vi "Main.vi"(11 "Module Admin":refnum<class "Delacor_lib_QMH_Module Admin.lvclass">) -> ()   [LabVIEW 2019, in "Panther Dashboard.lvlib"]
doc: "Panther Dashboard For DQMH®\n\nDeveloped and maintained by:\nPantherLAB\n\nMain Contributor- Developer:\n\n» Enrique Noé Arias\n\nBrainstorming & Code Reviews:\n\n» Matthias Baudot\n» Fabiola De La Cueva\n» Christopher Farmer\n» Cyril Gambini\n» Joerg Hampel\n» Olivier Jourdan\n» Cesar Muñoz\n» Darren Nattinger\n» Luis Orozco\n» Sam Taggart\n» Diego Torres"
uses:
  Panther Dashboard.lvlib
  <vilib>/Delacor/Delacor QMH/Libraries/Module Admin_class/Delacor_lib_QMH_Module Admin.lvclass
  Module Data--cluster.ctl
  Maps List and refs--cluster.ctl
  <vilib>/National Instruments/Tree Map/Tree Map Data.ctl
  DQMH Modules Info--cluster.ctl
  Module type--enum.ctl
  Project References--cluster.ctl
  Selection Type--enum.ctl
  References Updated Argument--cluster.ctl
  Launch DQMH Scripting Tools Argument--cluster.ctl
  DQMH Tools Menu--enum.ctl
  <vilib>/Delacor/Delacor QMH/Libraries/Message Queue_class/Delacor_lib_QMH_Message Queue.lvclass/Delacor_lib_QMH_Message Queue.ctl
  Expand Results Argument--cluster.ctl
  Execute Default Event Request Argument--cluster.ctl
  Tree DQMH Selection Argument--cluster.ctl
  Scan DQMH Modules Argument--cluster.ctl
  Stop Argument--cluster.ctl
  Generate Project Documentation Argument--cluster.ctl
  Set App Theme Argument--cluster.ctl
  Show About Argument--cluster.ctl
  Update Module ID Argument--cluster.ctl
  Save Library Description Argument--cluster.ctl
  Save VI Description Argument--cluster.ctl
  Open Documentation Argument--cluster.ctl
  Save Project Documentation Argument--cluster.ctl
  <vilib>/Delacor/Delacor QMH/Libraries/Module Admin_class/Delacor_lib_QMH_Module Admin.lvclass/Delacor_lib_QMH_Module Admin.ctl
  <vilib>/Delacor/Delacor QMH/Libraries/Message Queue_class/Delacor_lib_QMH_Enqueue Message (Single).vi
  <vilib>/Delacor/Delacor QMH/Libraries/Module Admin_class/Delacor_lib_QMH_Get External Launch.vi
  Panther Dashboard--global.vi
  <vilib>/National Instruments/Tree Map/API/List Roots.vi
  <vilib>/National Instruments/Tree Map/Utility/Into Tree Control Items.vi
  <vilib>/Platform/browser.llb/Open URL in Default Browser (path).vi
  <vilib>/Utility/error.llb/Error Cluster From Error Code.vi
  <vilib>/ErrorRing/Error Ring.xnode
  <vilib>/Delacor/Delacor QMH/Libraries/Message Queue_class/Delacor_lib_QMH_Message Queue.lvclass
  <vilib>/National Instruments/Tree Map/Tree Map.lvlib
  <vilib>/Delacor/Delacor QMH/Libraries/Scripting API/DQMH_Scripting API.lvlib
  Shared/Shared.lvlib
  ContextHelp/ContextHelp.lvlib
panel:
  out "error out":errorcluster
  in  "Add Event":bool
  in  "Remove Event":bool caption="Remove"
  in  "Convert Event":bool caption="Convert"
  in  "Rename Event":bool caption="Rename"
  in  "Add New Module":bool caption="Add"
  in  "Rename Module":bool caption="Rename"
  in  "Validate Module":bool caption="Validate"
  in  "Create Module Template":bool caption="Template"
  in  "Add Unit Test Module":bool caption="Unit Test"
  in  "Create RT Tester Module":bool caption="RT Tester"
  in  "Open Antidoc Output":bool caption="Open"
  in  "Generate Antidoc":bool caption="Antidoc"
  in  "About Panther":bool caption="About"
  in  "Theme Panther":bool caption="Theme"
  in  "Projects":string(combo)
  in  "Targets":string(combo)
  in  "Doc Editor":bool
  in  "Search":bool caption="Scan Project"
  in  "Expand Results":bool
  in  "Include Dependencies":bool
  in  "Module ID":i32=-1 min=-1 max=1000 step=1 format="Module ID %d"
  in  "Modules Tree":string(tree) caption="Tree 2"
  out "antidoc":bool
  out "Panther Indicator":bool
  out "Process Indicator":bool
  out "Event Indicator":bool
  out "Status":string
  out "Progress":u16(slide) scale=0.0..1.0
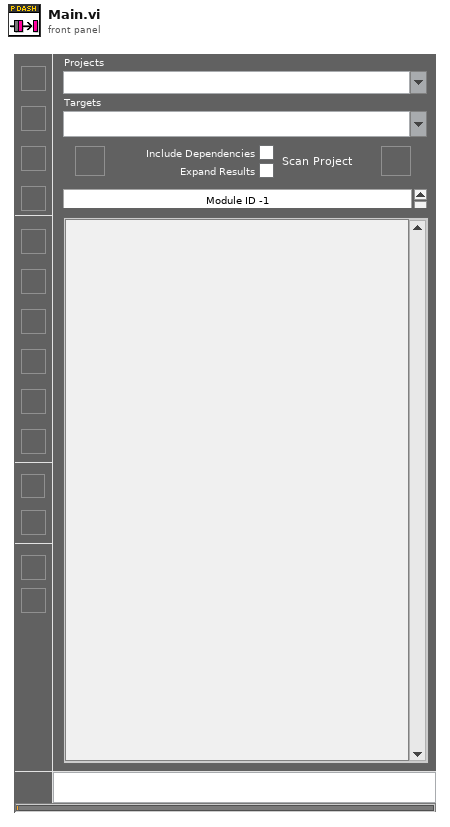
[diagram p1: front panel]
types:
  T1 = typedef "Panther Dashboard.lvlib/Broadcast Events--cluster.ctl" = cluster{"Module Did Init":refnum<user-event>, "Status Updated":refnum<user-event>, "Error Reported":refnum<user-event>, "Module Did Stop":refnum<user-event>, "Update Module Execution Status":refnum<user-event>, "References Updated":refnum<user-event>, "Projects Updated":refnum<user-event>, "Targets Updated":refnum<user-event>, "Progress updated":refnum<user-event>, "Scale Updated":refnum<user-event>, "Connector Pane Updated":refnum<user-event>, "Documentation Updated":refnum<user-event>, "Module Type Updated":refnum<user-event>, "Theme Updated":refnum<user-event>, "Project Description Updated":refnum<user-event>}
  T2 = typedef "Panther Dashboard.lvlib/Request Events--cluster.ctl" = cluster{"Stop Module":refnum<user-event>, "Show Panel":refnum<user-event>, "Hide Panel":refnum<user-event>, "Get Module Execution Status":refnum<user-event>, "Show Diagram":refnum<user-event>, "Scan DQMH Modules":refnum<user-event>, "Tree DQMH Selection":refnum<user-event>, "Open Module API Tester":refnum<user-event>, "Execute Default Event Request":refnum<user-event>, "Expand Results":refnum<user-event>, "Launch DQMH Scripting Tools":refnum<user-event>, "Generate Project Documentation":refnum<user-event>, "Set App Theme":refnum<user-event>, "Show About":refnum<user-event>, "Update Module ID":refnum<user-event>, "Save Library Description":refnum<user-event>, "Save VI Description":refnum<user-event>, "Open Documentation":refnum<user-event>, "Save Project Documentation":refnum<user-event>, "Register controls Mouse Enter":refnum<user-event>}
  T3 = typedef "ContextHelp.lvlib/Broadcast Events--cluster.ctl" = cluster{"Module Did Init":refnum<user-event>, "Status Updated":refnum<user-event>, "Error Reported":refnum<user-event>, "Module Did Stop":refnum<user-event>, "Update Module Execution Status":refnum<user-event>}
  T4 = typedef "Panther Dashboard.lvlib/Selection Type--enum.ctl" = enum16{"Broadcast", "Request", "Module", "Public API"}
  T5 = typedef "Panther Dashboard.lvlib/Module Data--cluster.ctl" = cluster{"Maps":T6, "DQMH Scan Results":T8, "Current Selection":cluster{"VI Ref":refnum<vi>, "DQMH Lib Ref":refnum<vi>}, "Module type":T9, "Module ID":i32, "Theme":bool, "Broadcast?":bool}
  T6 = typedef "Panther Dashboard.lvlib/Maps List and refs--cluster.ctl" = cluster{"Tree Map":T7, "References Map":map{string, refnum<vi>}}
  T7 = typedef "Tree Map.lvlib/Tree Map Data.ctl" = map{string, cluster{"Child Paths Set":set{string}, "Name":string, "Data":string, "Attributes":map{string, string}}}
  T8 = typedef "Panther Dashboard.lvlib/DQMH Modules Info--cluster.ctl" = cluster{"All DQMH Modules Refs":refnum<vi>[], "All Modules Descriptions":string[], "All Modules type":T9[], "Project References":T10}
  T9 = typedef "Panther Dashboard.lvlib/Module type--enum.ctl" = enum16{"Module type: Singleton", "Module type: Cloneable"}
  T10 = typedef "Panther Dashboard.lvlib/Project References--cluster.ctl" = cluster{"Project Ref":refnum<vi>, "Project Name":string, "Target":refnum<vi>, "App Ref":refnum<vi>}
  T11 = typedef "Panther Dashboard.lvlib/References Updated Argument--cluster.ctl" = cluster{"Modules":refnum<vi>[], "Modules Types":T9[], "Application Instance":refnum<vi>}
  T12 = enum8{"Enabled", "Disabled", "Disabled and Grayed Out"}
  T13 = typedef "Panther Dashboard.lvlib/Launch DQMH Scripting Tools Argument--cluster.ctl" = cluster{"Scripting Tool":T14}
  T14 = typedef "Panther Dashboard.lvlib/DQMH Tools Menu--enum.ctl" = enum16{"Create New DQMH Event", "Remove DQMH Event", "Convert DQMH Event", "Rename DQMH Event", "Add New DQMH Module", "Create RT Tester", "Rename DQMH Module", "Validate DQMH Module", "Create DQMH Module Template", "New DQMH  Unit Test"}
  T15 = typedef "Panther Dashboard.lvlib/Expand Results Argument--cluster.ctl" = cluster{"Expand?":bool}
  T16 = typedef "Panther Dashboard.lvlib/Execute Default Event Request Argument--cluster.ctl" = cluster{"Event Name":string}
  T17 = typedef "Panther Dashboard.lvlib/Tree DQMH Selection Argument--cluster.ctl" = cluster{"Tree DQMH Sel":string}
  T18 = typedef "Panther Dashboard.lvlib/Scan DQMH Modules Argument--cluster.ctl" = cluster{"Include Dependencies":bool, "Project":string, "Target":string}
  T19 = enum32{"invalid lock state", "Not Locked", "Locked (No Password)", "Password-protected"}
  T20 = typedef "Panther Dashboard.lvlib/Stop Argument--cluster.ctl" = cluster{"Origin":string, "Exit via Stop Module Req?":bool, "Wait for Module to stop?":bool}
  T21 = typedef "Panther Dashboard.lvlib/Generate Project Documentation Argument--cluster.ctl" = cluster{"Boolean":bool}
  T22 = typedef "Panther Dashboard.lvlib/Set App Theme Argument--cluster.ctl" = cluster{"Theme":bool}
  T23 = typedef "Panther Dashboard.lvlib/Show About Argument--cluster.ctl" = cluster{"Boolean":bool}
  T24 = typedef "Panther Dashboard.lvlib/Update Module ID Argument--cluster.ctl" = cluster{"New ID":i32}
  T25 = typedef "Panther Dashboard.lvlib/Save Library Description Argument--cluster.ctl" = cluster{"Library Description":string}
  T26 = typedef "Panther Dashboard.lvlib/Save VI Description Argument--cluster.ctl" = cluster{"VI Description":string}
  T27 = typedef "Panther Dashboard.lvlib/Open Documentation Argument--cluster.ctl" = cluster{"Boolean":bool}
  T28 = typedef "Panther Dashboard.lvlib/Save Project Documentation Argument--cluster.ctl" = cluster{"Project Description":string}
  T29 = cluster{"Left Cell String":string, "Child Text":string[], "Child Tag":string, "Item Indent":i32, "Child Only?":bool, "Glyph Index":i32}[]
  T30 = typedef "LVRectTypeDef.ctl" = cluster{"Left":i16, "Top":i16, "Right":i16, "Bottom":i16}
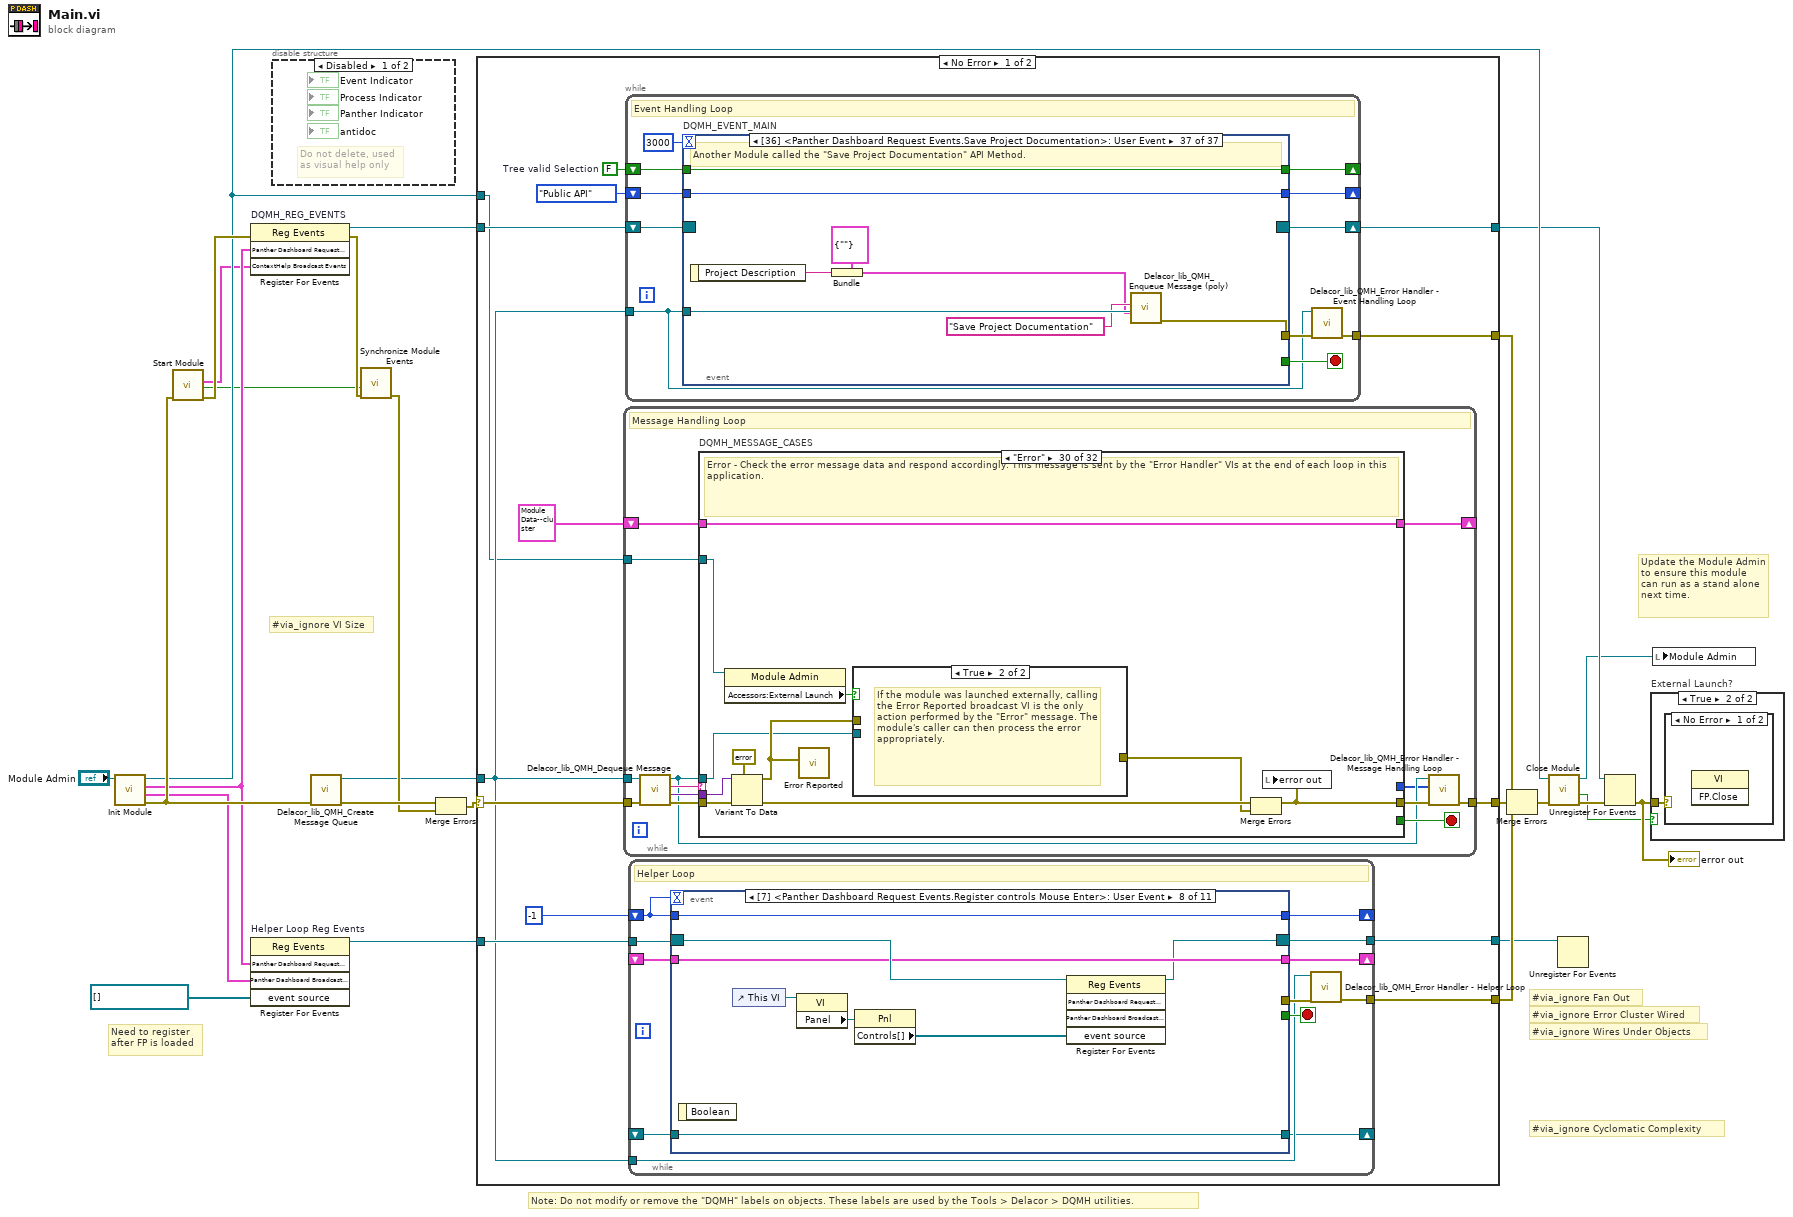
[diagram p0: block diagram]
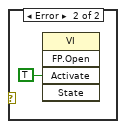
[diagram p4: hidden frame]
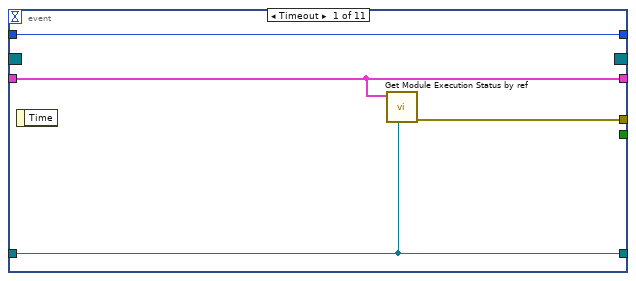
[diagram p5: hidden frame]
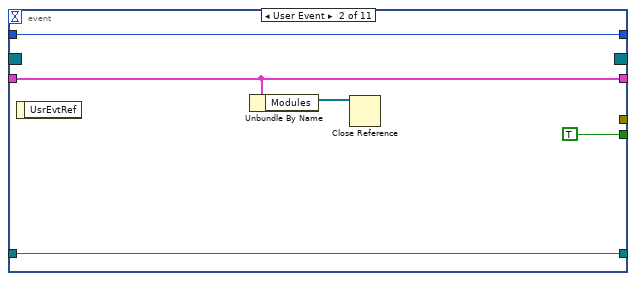
[diagram p6: hidden frame]
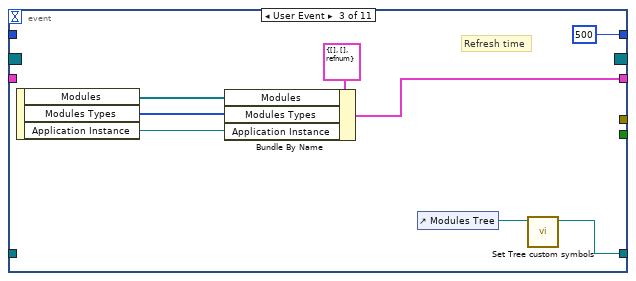
[diagram p7: hidden frame]
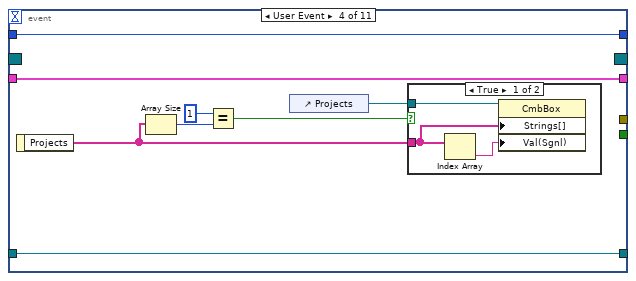
[diagram p8: hidden frame]
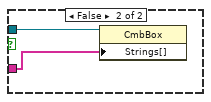
[diagram p9: hidden frame]
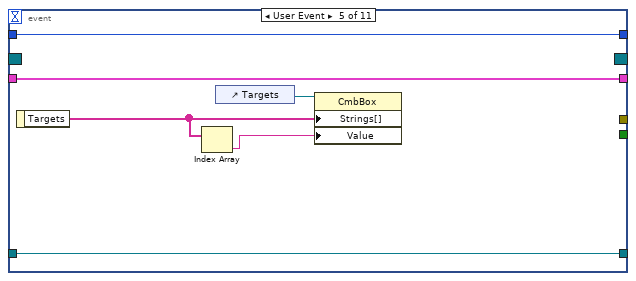
[diagram p10: hidden frame]
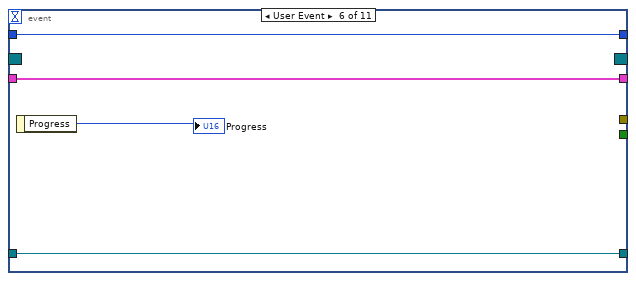
[diagram p11: hidden frame]
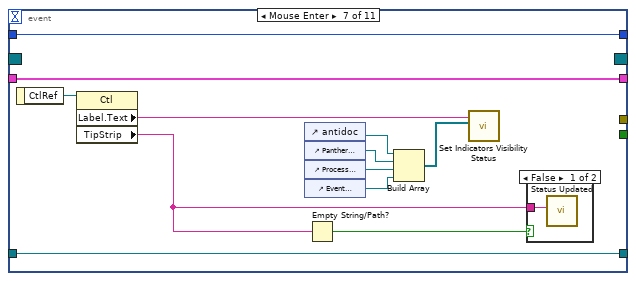
[diagram p12: hidden frame]
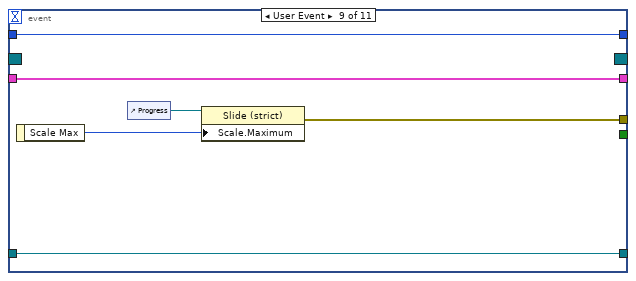
[diagram p14: hidden frame]
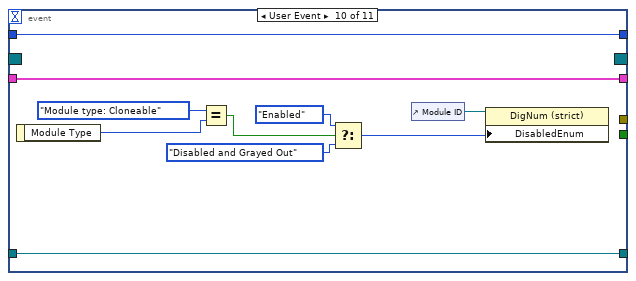
[diagram p15: hidden frame]
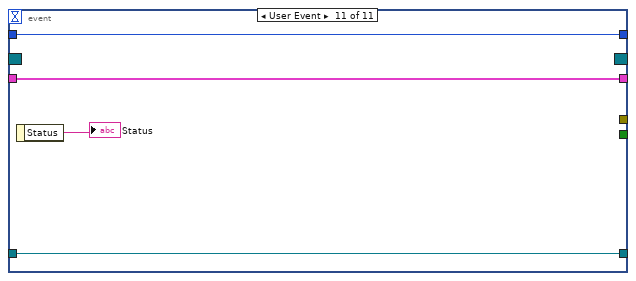
[diagram p16: hidden frame]
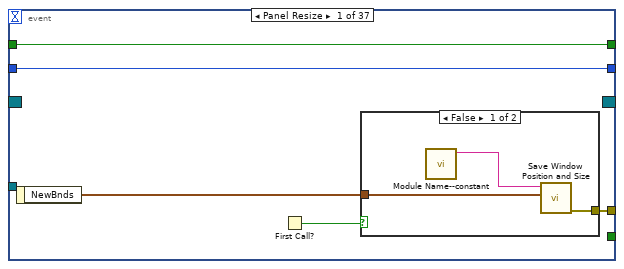
[diagram p17: hidden frame]
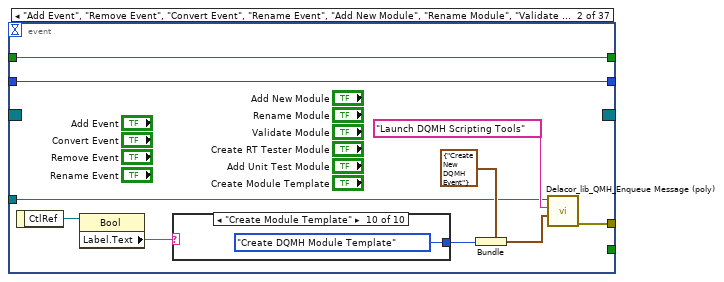
[diagram p19: hidden frame]
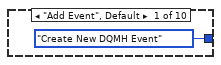
[diagram p20: hidden frame]
diagram:
  # "Need to register\nafter FP is loaded"
  # "#via_ignore VI Size"
  # "#via_ignore Fan Out"
  # "#via_ignore Cyclomatic Complexity"
  # "#via_ignore Wires Under Objects"
  # "#via_ignore Error Cluster Wired"
  # "Note: Do not modify or remove the \"DQMH\" labels on objects. These labels are used by the Tools > Delacor > DQMH utilities."
  # "Update the Module Admin to ensure this module can run as a stand alone next time."
  n1 = call "Init Module.vi"("Singleton Module Admin in"="Module Admin") -> ("error out"=w15:errorcluster, "Panther Dashboard Broadcast Events"=w4:T1, "Panther Dashboard Request Events"=w5:T2, "Singleton Module Admin out"=w14:refnum<class "Delacor_lib_QMH_Module Admin.lvclass">)  [unwired: 7 in]
  n2 = call "Start Module.vi"("error in"=w15) -> ("error out"=w17:errorcluster, "Wait for Event Sync?"=w3:bool, "ContextHelp Broadcast Events"=w2:T3)  [unwired: 7 in, 1 out]
  n3 = register-events "DQMH_REG_EVENTS"(error in=w17, w5, w2) -> (reference out=w12:refnum<event-registration>, error out=w18:errorcluster)  [unwired: 1 in]
  n4 = register-events "Helper Loop Reg Events"(w5, w4, refnum<vi>[] [] ("event source")) -> (reference out=w7:refnum<event-registration>)  [unwired: 2 in, 1 out]
  n5 = disable-structure shown="Disabled" {
    frame Disabled {
      # "Do not delete, used\nas visual help only"
    }
    frame Enabled {
    }
  }
  n6 = call <vilib>:"Delacor_lib_QMH_Create Message Queue.vi"("error in"=w15) -> ("error out"=w21:errorcluster, "Message Queue"=w11:refnum<class "Delacor_lib_QMH_Message Queue.lvclass">)  [unwired: 9 in]
  n7 = call "Synchronize Module Events.vi"("error in"=w18, "Wait for Event Sync?"=w3) -> ("error out"=w16:errorcluster)  [unwired: 9 in]
  n8 = Merge Errors(w21, w16) -> (w20:errorcluster)
  n9 = case shown="No Error" w20 {
    selector: w20 -> [w38 w815]
    tunnel: [w40 w814] -> w26
    tunnel: [w36 w813] -> w13
    tunnel: w12 -> [w34 w813]
    tunnel: w11 -> [w30 w809]
    tunnel: [w39 _] -> w24
    tunnel: w14 -> [w27 w810]
    tunnel: w7 -> [w33 w808]
    tunnel: [w32 w808] -> w6
    tunnel: [w37 _] -> w19
    frame No Error {
      w29 = FALSE  # Tree valid Selection
      n10 = while {
        tunnel: w30 -> [w458]
        shift-right: [w462] -> _
        shift-left: T5 {"Maps"={"Tree Map"={}, "References Map"={}}, "DQMH Scan Results"={"All DQMH Modules Refs"=[], "All Modules Descriptions"=[], "All Modules type"=[], "Project References"={"Project Ref"=refnum, "Project Name"="", "Target"=refnum, "App Ref"=refnum}}, "Current Selection"={"VI Ref"=refnum, "DQMH Lib Ref"=refnum}, "Module type"=enum."Module type: Singleton", "Module ID"=0, "Theme"=FALSE, "Broadcast?"=FALSE} ("Data Cluster") -> [w463]
        tunnel: w38 -> [w466]
        tunnel: [w464] -> w40
        tunnel: w27 -> [w456]
        stop <- w461 stop-if-true
        # "Message Handling Loop"
        n11 = call-dynamic "Delacor_lib_QMH_Dequeue Message.vi"("error in"=w466, "Message Queue in"=w458) -> ("error out"=w465:errorcluster, "Message Data"=w459:variant, "Message"=w460:string, "Message Queue out"=w457:refnum<class "Delacor_lib_QMH_Message Queue.lvclass">)  [unwired: 6 in]
        n12 = case "DQMH_MESSAGE_CASES" shown="\"Error\"" w460 {
          selector: w460 -> [_ w491 _ _ _ _ _ _ _ _ _ _ _ _ _ _ _ _ _ _ _ _ _ _ _ _ _ _ _ _ _ w794]
          tunnel: w457 -> [_ _ _ _ _ _ _ _ _ _ _ _ _ _ _ _ _ _ _ _ _ _ _ _ _ _ _ _ _ w760 w786 _]
          tunnel: w465 -> [w488 w496 w498 w519 w526 w533 w540 w555 w564 w569 w575 w589 w602 w624 w630 w637 w644 w649 w662 w671 w682 w691 w699 w709 w725 w741 w752 w755 w757 w767 w792 w796]
          tunnel: [w482 w494 w498 w518 w525 w533 w540 w554 w563 w570 w576 w587 w600 w625 w629 w636 w643 w648 w660 w669 w672 w687 w698 w707 w723 w740 w750 w754 w757 w763 w789 w797] -> w467
          tunnel: w463 -> [w479 w493 w497 w505 w523 w531 w539 w550 w562 w568 w574 w582 w599 w623 w628 w635 w642 w647 w651 w665 w679 w686 w697 w701 w718 w730 w746 w753 w756 w762 w778 w795]
          tunnel: [w478 w493 w497 w510 w523 w531 w539 w546 w562 w568 w574 w582 w599 w623 w628 w633 w642 w647 w651 w665 w674 w686 w693 w700 w716 w730 w746 w753 w756 w762 w778 w795] -> w462
          tunnel: [_ _ _ _ _ _ _ _ _ _ _ _ _ _ _ _ _ _ _ _ _ _ _ _ _ _ _ _ _ _ w785 _] -> w461
          tunnel: w459 -> [_ w492 _ w513 _ _ _ w553 _ _ _ w585 _ _ _ w634 w641 _ w659 w667 w678 w685 w696 w705 w721 w739 w749 _ _ w761 w784 _]
          tunnel: w456 -> [w480 _ _ _ _ _ _ _ _ _ _ _ _ _ _ _ _ _ _ _ _ _ _ _ _ _ _ _ _ w759 w779 _]
          tunnel: [_ _ _ _ _ _ _ _ _ _ _ _ i32[] [5000, 1026, 43] ("specific error code to clear (0: all)") _ _ _ _ _ _ _ _ _ _ _ _ _ _ _ _ _ _ _] -> w455
          frame "Initialize" {
            w469 = "Panther Dashboard for DQMH" ("format string")
            # "Initialize - Any operation that needs to be done before the module can receive messages. Synchronize Caller Events.vi will inform Start Module.vi that the module has launched and is ready to receive messages. Module Did Init.vi will broadcast that the module initialized."
            n13 = call "Synchronize Caller Events.vi"("error in (no error)"=w488, "Singleton Module Admin in"=w480) -> ("error out"=w487:errorcluster)  [unwired: 8 in, 1 out]
            n14 = invoke on="Modules Tree" class="Tree (strict)" method="Edit Tree Items.Delete"() -> ()  [unwired: 5 in, 5 out]
            n15 = property on="Modules Tree" class="Tree (strict)"("Allow Item Drag"=TRUE ("Drag/Drop:Allow Dragging"), "SelColor"=u32 8355711) -> ()  [unwired: 2 in, 2 out]
            n16 = call "Module Name--constant.vi"() -> ("Module Name"=w476:string)  [unwired: 11 in]
            n17 = call "Module Did Init.vi"("error in (no error)"=w487, "Initialized?"=TRUE, "Origin"=w476) -> ("error out"=w486:errorcluster)  [unwired: 8 in]
            n18 = control-ref of="Projects"() -> (w472:refnum<vi>)
            n19 = call "Scan For App Projects.vi"("error in"=w486, "Init?"=TRUE, "Projects Ref"=w472) -> ("error out"=w485:errorcluster)  [unwired: 8 in]
            n20 = call "Read Theme from Config.vi"("error in"=w485) -> ("error out"=w484:errorcluster, "Theme"=w468:bool)  [unwired: 9 in]
            n21 = local write "Theme Panther"(w468) -> ()
            n22 = call "Set App Theme.vi"("error in"=w484, "Theme"=w468) -> ("error out"=w483:errorcluster)  [unwired: 9 in]
            n23 = control-ref of="This VI"() -> (w470:refnum<vi>)
            n24 = Bundle By Name(cluster=w479, "Module ID"=-1) -> (w478:T5)
            n25 = call "Status Updated.vi"("Status"=w469) -> ()  [unwired: 10 in, 1 out]
            n26 = call "Set Panel Initial State.vi"("Title"=w469, "Main Vi Ref"=w470) -> ("error out"=w481:errorcluster)  [unwired: 9 in]
            n27 = Merge Errors(w481, w483) -> (w482:errorcluster)
          }
          frame "Refresh Targets" {
            # "When the User selects a Project triggers this task to scan all the targets available"
            n28 = Variant To Data(error in=w496, type=w491, Variant=w492) -> (data=w490:string, error out=w495:errorcluster)
            n29 = call "Get all Targets.vi"("error in"=w495, "Project Selection"=w490) -> ("error out"=w494:errorcluster, "Targets"=w489:string[])  [unwired: 8 in]
            n30 = call "Targets Updated.vi"("Targets"=w489) -> ()  [unwired: 10 in, 1 out]
          }
          frame "---Module Specific---" {
            # "Separator -- The following cases handle messages specific to this Module."
          }
          frame "Scan DQMH Modules" {
            # "Scan DQMH Modules in the project and fill 2 maps one with the Vi References and the another one with the list of DQMH modules on the project"
            n31 = Variant To Data(error in=w519, type=T18 {"Include Dependencies"=FALSE, "Project"="", "Target"=""} ("Scan DQMH Modules Argument"), Variant=w513) -> (data=w511:T18, error out=w516:errorcluster)
            n32 = call "Close vi references.vi"("Data Cluster"=w505) -> ("error out"=w515:errorcluster)  [unwired: 10 in]
            n33 = Unbundle By Name(w511) -> ("Project"=w501:string, "Target"=w503:string, "Include Dependencies"=w504:bool)
            n34 = invoke on="Modules Tree" class="Tree (strict)" method="Edit Tree Items.Delete"(error in=w515, "Delete Children"=TRUE ("Delete Children?")) -> (error out=w514:errorcluster)  [unwired: 3 in, 4 out]
            n35 = local write "Include Dependencies"(w504) -> ()
            n36 = call <vilib>:"Set Busy.vi"("error in (no error)"=w514) -> ()  [unwired: 9 in, 2 out]
            n37 = call "Scan DQMH Modules and create Maps.vi"("error in"=w516, "Include Dependencies"=w504, "Target Selection"=w503, "Project"=w501) -> ("error out"=w518:errorcluster, "Tree Map out"=w502:T7, "map ref out"=w506:map{string, refnum<vi>}, "DQMH Scan Results"=w509:T8)  [unwired: 4 in]
            n38 = control-ref of="Modules Tree"() -> (w507:refnum<vi>)
            n39 = call <vilib>:"Tree Map to Tree Control Items.vi"("Tree Map In"=w502) -> ("Tree Control Items"=w508:T29)  [unwired: 10 in]
            n40 = Bundle By Name(cluster=w505, "DQMH Scan Results"=w509, "Maps.References Map"=w506, "Maps.Tree Map"=w502) -> (w510:T5)
            n41 = local read "Expand Results"() -> (w499:bool)
            n42 = call "Draw Tree.vi"("Expanded Results?"=w499, "Tree Control Items"=w508, "TreeControl in"=w507) -> ("error out"=w517:errorcluster)  [unwired: 8 in]
            n43 = call <vilib>:"Unset Busy.vi"("error in (no error)"=w517) -> ()  [unwired: 10 in, 1 out]
          }
          frame "Drag VI" {
            # "This is the functionality alowing drag and drop the current selection to your code, you can build code using panther Dashboard."
            n44 = Unbundle By Name(w523) -> ("DQMH Scan Results.Project References.App Ref"=w522:refnum<vi>, "DQMH Scan Results.Project References.Target"=w521:refnum<vi>, "Current Selection.VI Ref"=w520:refnum<vi>)
            n45 = call "Drop Event into subVI.vi"("Current Selection.VI Ref"=w520, "Target"=w521, "App Ref"=w522) -> ("error out"=w524:errorcluster)  [unwired: 8 in]
            n46 = Merge Errors(w524, w526) -> (w525:errorcluster)
          }
          frame "Who is launching this module?" {
            w532 = 0  # Start Module.vi index
            # "Find all the VIS calling the Start Module.vi of the selected module library"
            n47 = Unbundle By Name(w531) -> ("Theme"=w530:bool, "DQMH Scan Results.Project References.App Ref"=w529:refnum<vi>, "DQMH Scan Results.Project References.Target"=w528:refnum<vi>, "Current Selection.DQMH Lib Ref"=w527:refnum<vi>)
            n48 = call "Find some Public API VI.vi"("Theme"=w530, "Public Api file index"=w532, "Library in"=w527, "Target"=w528, "App Ref"=w529) -> ()  [unwired: 7 in]
          }
          frame "Who is registered to this module's broadcasts?" {
            w538 = 2  # Obtain Broadcast Events for Registration.vi index
            # "Find all the VIS calling the Obtain broadcast events for registration of the selected module library"
            n49 = Unbundle By Name(w539) -> ("Theme"=w537:bool, "DQMH Scan Results.Project References.App Ref"=w536:refnum<vi>, "DQMH Scan Results.Project References.Target"=w535:refnum<vi>, "Current Selection.DQMH Lib Ref"=w534:refnum<vi>)
            n50 = call "Find some Public API VI.vi"("Theme"=w537, "Public Api file index"=w538, "Library in"=w534, "Target"=w535, "App Ref"=w536) -> ()  [unwired: 7 in]
          }
          frame "Tree DQMH Selection" {
            # "There is a new selection of the DQMH Tree list, need to search and update indicators acordanly."
            n51 = Unbundle By Name(w550) -> ("Maps.Tree Map"=w549:T7, "Maps.References Map"=w548:map{string, refnum<vi>}, "DQMH Scan Results"=w547:T8)
            n52 = Variant To Data(error in=w555, type=T17 {"Tree DQMH Sel"=""} ("Tree DQMH Selection Argument"), Variant=w553) -> (data=w551:T17, error out=w554:errorcluster)
            n53 = Unbundle By Name(w551) -> ("Tree DQMH Sel"=w543:string)
            n54 = call "Get List Information.vi"("List Selection"=w543, "DQMH Scan Info"=w547, "References Map"=w548, "Tree Map"=w549) -> ("Broadcast?"=w541:bool, "Vi out"=w544:refnum<vi>, "Module type"=w542:T9, "DQMH Lib"=w545:refnum<vi>)  [unwired: 4 in]
            n55 = Bundle By Name(cluster=w550, "Current Selection.DQMH Lib Ref"=w545, "Current Selection.VI Ref"=w544, "Module type"=w542, "Broadcast?"=w541) -> (w546:T5)
          }
          frame "Open Module API Tester" {
            # "If nothing selected use the first DQMH module"
            # "Open the API Tester from the current DQMH Module Selected"
            n56 = Unbundle By Name(w562) -> ("DQMH Scan Results.Project References.App Ref"=w561:refnum<vi>, "DQMH Scan Results.All DQMH Modules Refs"=w560:refnum<vi>[], "Current Selection.DQMH Lib Ref"=w556:refnum<vi>)
            n57 = Index Array(array=w560) -> (element=w558:refnum<vi>)  [unwired: 1 in]
            n58 = Not A Number/Path/Refnum?(number/path/refnum=w556) -> (NaN/Path/Refnum?=w559:bool)
            n59 = Select(t=w558, s=w559, f=w556) -> (s? t:f=w557:refnum<vi>)
            n60 = call "Open API Tester.vi"("error in"=w564, "DQMH Library Ref"=w557, "Application Instance"=w561) -> ("error out"=w563:errorcluster)  [unwired: 8 in]
          }
          frame "Find Module in project" {
            # "Find the selected module in project explorer"
            n61 = Unbundle By Name(w568) -> ("Current Selection.DQMH Lib Ref"=w567:refnum<vi>, "DQMH Scan Results.Project References.Project Ref"=w566:refnum<vi>, "DQMH Scan Results.All DQMH Modules Refs"=w565:refnum<vi>[])
            n62 = call "Find Library in Project.vi"("error in (no error)"=w569, "DQMH Modules Refs"=w565, "Project Ref"=w566, "DQMH Lib Ref"=w567) -> ("error out"=w570:errorcluster)  [unwired: 7 in]
          }
          frame "Locate Event on Main" {
            # "Find the selected event vi on the owing DQMH Module, if it is a reques we highlight its frame, if it is a broadcast we highlight where the broadcast is being triggered"
            n63 = Unbundle By Name(w574) -> ("DQMH Scan Results.Project References.App Ref"=w572:refnum<vi>, "Current Selection.VI Ref"=w573:refnum<vi>, "Broadcast?"=w571:bool)
            n64 = call "Find Event Frame.vi"("error in"=w575, "Broadcast?"=w571, "VI in"=w573, "Application Instance"=w572) -> ("error out"=w576:errorcluster)  [unwired: 7 in]
          }
          frame "Execute Default Event Request" {
            # "Execute Default Event"
            n65 = Variant To Data(error in=w589, type=T16 {"Event Name"=""} ("Execute Default Event Request Argument"), Variant=w585) -> (data=w583:T16, error out=w588:errorcluster)
            n66 = Unbundle By Name(w582) -> ("DQMH Scan Results.Project References.App Ref"=w581:refnum<vi>, "Current Selection.DQMH Lib Ref"=w580:refnum<vi>, "Module ID"=w578:i32, "Module type"=w577:T9)
            n67 = Unbundle By Name(w583) -> ("Event Name"=w579:string)
            n68 = call "Execute Default event.vi"("Module type"=w577, "Module ID"=w578, "Event"=w579, "DQMH Library Ref"=w580, "application Instance"=w581) -> ("error out"=w586:errorcluster)  [unwired: 6 in]
            n69 = Merge Errors(w588, w586) -> (w587:errorcluster)
          }
          frame "Search for Event Callers / listeners" {
            # "1026-Invalid Ref\n43- Operation\n canceled by user\n5000- something\nrandom happening\non DQMH Scripting\nAPI"
            # "Search for this event callers"
            n70 = Unbundle By Name(w599) -> ("DQMH Scan Results.Project References.Project Ref"=w593:refnum<vi>, "Current Selection.VI Ref"=w598:refnum<vi>, "Theme"=w590:bool, "Broadcast?"=w591:bool)
            n71 = Select(t="Searching code registered to broadcast selection" ("Status"), s=w591, f="Searching for Event Callers" ("Status")) -> (s? t:f=w594:string)
            n72 = call "Status Updated.vi"("error in (no error)"=w602, "Status"=w594) -> ("error out"=w601:errorcluster)  [unwired: 9 in]
            n73 = case shown="False" w591 {
              tunnel: w601 -> [w607 w614]
              tunnel: [w606 w613] -> w600
              tunnel: w598 -> [w605 w610]
              tunnel: [w604 w612] -> w597
              tunnel: w593 -> [w603 w611]
              frame False {
                # "Requests"
                n74 = call <vilib>:"Get Callers of Request VI in Project.vi"("error in"=w607, "Request VI"=w605, "Project"=w603) -> ("error out"=w606:errorcluster, "Request VI Callers"=w604:refnum<vi>[])  [unwired: 7 in]
              }
              frame True {
                # "Broadcast"
                n75 = Two Button Dialog(message="This is an exhaustive task that can take up to minutes, do you wish to continue?") -> (T button?=w609:bool)  [unwired: 2 in]
                n76 = case shown="False" w609 {
                  tunnel: w614 -> [w615 w620]
                  tunnel: [w615 w619] -> w613
                  tunnel: [_ w618] -> w612
                  tunnel: w611 -> [_ w617]
                  tunnel: w610 -> [_ w616]
                  frame False {
                  }
                  frame True {
                    n77 = call <vilib>:"Get VIs Registered for Broadcast in Project.vi"("error in"=w620, "Broadcast VI"=w616, "Project"=w617) -> ("error out"=w619:errorcluster, "VIs Registered for Broadcast"=w618:refnum<vi>[])  [unwired: 7 in]
                  }
                }
              }
            }
            n78 = call <vilib>:"Set Busy.vi"("error in (no error)"=w601) -> ()  [unwired: 9 in, 2 out]
            n79 = call <vilib>:"Unset Busy.vi"("error in (no error)"=w600) -> ()  [unwired: 10 in, 1 out]
            n80 = call "Start Call to results window.vi"("Find Broadcast?"=w591, "Request VI Callers"=w597, "Event"=w598, "Theme"=w590) -> ()  [unwired: 8 in]
          }
          frame "Open VI on Disk" {
            # "Open current event selection on the file system"
            n81 = Unbundle By Name(w623) -> ("Current Selection.VI Ref"=w622:refnum<vi>)
            n82 = property class="VI"(reference=w622) -> ("Path"=w621:path)  [unwired: 1 in, 2 out]
            n83 = call "Open File on Disk.vi"("error in"=w624, "file or directory path"=w621) -> ("error out"=w625:errorcluster)  [unwired: 9 in]
          }
          frame "Open File Library on Disk" {
            # "Open current Module Library selection on the file system"
            n84 = Unbundle By Name(w628) -> ("Current Selection.DQMH Lib Ref"=w627:refnum<vi>)
            n85 = property class="Library"(reference=w627) -> ("Path"=w626:path)  [unwired: 1 in, 2 out]
            n86 = call "Open File on Disk.vi"("error in"=w630, "file or directory path"=w626) -> ("error out"=w629:errorcluster)  [unwired: 9 in]
          }
          frame "Module ID Update" {
            # "Module ID Control has value change"
            n87 = Variant To Data(error in=w637, type=0 ("Module ID"), Variant=w634) -> (data=w632:i32, error out=w636:errorcluster)
            n88 = Bundle By Name(cluster=w635, "Module ID"=w632) -> (w633:T5)
          }
          frame "Expand or Close" {
            # "Expand or Close DQMH Tree control"
            n89 = Variant To Data(error in=w644, type=T15 {"Expand?"=FALSE} ("Expand or Close Argument"), Variant=w641) -> (data=w639:T15, error out=w643:errorcluster)
            n90 = Unbundle By Name(w639) -> ("Expand?"=w638:bool)
            n91 = invoke on="Modules Tree" class="Tree (strict)" method="Open/Close.Open/Close All"("Open"=w638) -> ()  [unwired: 3 in, 4 out]
          }
          frame "Open Project Folder" {
            n92 = Unbundle By Name(w647) -> ("DQMH Scan Results.Project References.Project Ref"=w646:refnum<vi>)
            n93 = property class="Project"(reference=w646) -> ("Path"=w645:path)  [unwired: 1 in, 2 out]
            n94 = call "Open File on Disk.vi"("error in"=w649, "file or directory path"=w645) -> ("error out"=w648:errorcluster)  [unwired: 9 in]
          }
          frame "Launch DQMH Scripting Tools" {
            # "Launch the DQMH Scripting Tools"
            n95 = Variant To Data(error in=w662, type=T13 {"Scripting Tool"=enum."Create New DQMH Event"} ("Launch DQMH Scripting Tools Argument"), Variant=w659) -> (data=w657:T13, error out=w661:errorcluster)
            n96 = Unbundle By Name(w657) -> ("Scripting Tool"=w652:T14)
            n97 = Unbundle By Name(w651) -> ("DQMH Scan Results.Project References.Project Name"=w655:string, "DQMH Scan Results.Project References.App Ref"=w656:refnum<vi>, "Current Selection.DQMH Lib Ref"=w650:refnum<vi>)
            n98 = Format Into String(format string="DQMH Tool: %s being executed ", w652) -> (resulting string=w654:string)  [unwired: 2 in, 1 out]
            n99 = call "Status Updated.vi"("Status"=w654) -> ()  [unwired: 10 in, 1 out]
            n100 = call "Launch DQMH Tools by menu.vi"("Project"=w655, "Application Instance"=w656, "error in"=w661, "Module Ref"=w650, "DQMH Tools"=w652) -> ("error out"=w660:errorcluster)  [unwired: 6 in]
          }
          frame "Generate Project Documentation" {
            n101 = Variant To Data(error in=w671, type=T21 {"Boolean"=FALSE} ("Generate Project Documentation Argument"), Variant=w667) -> (error out=w670:errorcluster)  [unwired: 1 out]
            n102 = Unbundle By Name(w665) -> ("DQMH Scan Results.Project References.Project Ref"=w664:refnum<vi>)
            n103 = property class="Project"(reference=w664) -> ("Path"=w663:path)  [unwired: 1 in, 2 out]
            n104 = call "Generate Documentation--dialog.vi"("Project Path"=w663) -> ("error out"=w668:errorcluster)  [unwired: 10 in]
            n105 = Merge Errors(w670, w668) -> (w669:errorcluster)
          }
          frame "Set App Theme" {
            # "Set Panther Dashboard Theme"
            n106 = Variant To Data(error in=w682, type=T22 {"Theme"=FALSE} ("Set App Theme Argument"), Variant=w678) -> (data=w676:T22, error out=w680:errorcluster)
            n107 = Unbundle By Name(w676) -> ("Theme"=w673:bool)
            n108 = control-ref of="This VI"() -> (w675:refnum<vi>)
            n109 = Bundle By Name(cluster=w679, "Theme"=w673) -> (w674:T5)
            n110 = call "Set Theme.vi"("Dark?"=w673, "VI in"=w675) -> ()  [unwired: 10 in]
            n111 = call "Theme Updated.vi"("Theme"=w673) -> ()  [unwired: 10 in, 1 out]
            n112 = call "Save Theme in config.vi"("error in"=w680, "Theme"=w673) -> ("error out"=w681:errorcluster)  [unwired: 9 in]
            n113 = call "Register controls Mouse Enter.vi"("error in"=w681) -> ("error out"=w672:errorcluster)  [unwired: 10 in]
          }
          frame "Show About" {
            # "Show About project"
            n114 = Variant To Data(error in=w691, type=T23 {"Boolean"=FALSE} ("Show About Argument"), Variant=w685) -> (error out=w688:errorcluster)  [unwired: 1 out]
            n115 = control-ref of="This VI"() -> (w683:refnum<vi>)
            n116 = call "Hide VI Panel.vi"("error in (no error)"=w688, "VI"=w683) -> ("error out"=w690:errorcluster)  [unwired: 9 in]
            n117 = call "About Panther Dashboard.vi"("error in"=w690) -> ("error out"=w689:errorcluster)  [unwired: 10 in]
            n118 = call "Open VI Panel.vi"("error in (no error)"=w689, "VI"=w683) -> ("error out"=w687:errorcluster)  [unwired: 9 in]
          }
          frame "Update Module ID" {
            # "Update the Current Module ID"
            n119 = Variant To Data(error in=w699, type=T24 {"New ID"=-1} ("Update Module ID Argument"), Variant=w696) -> (data=w694:T24, error out=w698:errorcluster)
            n120 = Unbundle By Name(w694) -> ("New ID"=w692:i32)
            n121 = Bundle By Name(cluster=w697, "Module ID"=w692) -> (w693:T5)
          }
          frame "Save Library Description" {
            # "Save Library Description"
            n122 = Variant To Data(error in=w709, type=T25 {"Library Description"=""} ("Save Library Description Argument"), Variant=w705) -> (data=w703:T25, error out=w708:errorcluster)
            n123 = Unbundle By Name(w703) -> ("Library Description"=w702:string)
            n124 = in-place {
              in-place-border: w702 -> [w713]
              in-place-border: [w715] -> w706
              n125 = in-place-cluster #1(w701) -> ("Current Selection.DQMH Lib Ref"=w714:refnum<vi>, "DQMH Scan Results"=w711:T8)
              n126 = call "Save Library Documentation.vi"("New Description"=w713, "DQMH Modules Info In"=w711, "Library in"=w714) -> ("error out"=w715:errorcluster, "DQMH Modules Info Out"=w712:T8, "Lib out"=w710:refnum<vi>)  [unwired: 6 in]
              n127 = in-place-cluster #1("Current Selection.DQMH Lib Ref"=w710, "DQMH Scan Results"=w712) -> (w700:T5)
            }
            n128 = Merge Errors(w708, w706) -> (w707:errorcluster)
          }
          frame "Save VI Description" {
            # "Save Event Description"
            n129 = Variant To Data(error in=w725, type=T26 {"VI Description"=""} ("Save VI Description Argument"), Variant=w721) -> (data=w719:T26, error out=w724:errorcluster)
            n130 = Unbundle By Name(w719) -> ("VI Description"=w717:string)
            n131 = in-place {
              in-place-border: w717 -> [w728]
              in-place-border: [w729] -> w722
              n132 = in-place-cluster #2(w718) -> ("Current Selection.VI Ref"=w727:refnum<vi>)
              n133 = call "Save Event Description.vi"("Event Description"=w728, "Event Ref in"=w727) -> ("error out"=w729:errorcluster, "Event Ref out"=w726:refnum<vi>)  [unwired: 8 in]
              n134 = in-place-cluster #2("Current Selection.VI Ref"=w726) -> (w716:T5)
            }
            n135 = Merge Errors(w724, w722) -> (w723:errorcluster)
          }
          frame "Open Documentation" {
            # "Open Antidoc Documentation"
            n136 = Variant To Data(error in=w741, type=T27 {"Boolean"=FALSE} ("Open Documentation Argument"), Variant=w739) -> (error out=w740:errorcluster)  [unwired: 1 out]
            n137 = Unbundle By Name(w730) -> ("DQMH Scan Results.Project References.Project Ref"=w737:refnum<vi>)
            n138 = property class="Project"(reference=w737) -> ("Path"=w736:path)  [unwired: 1 in, 2 out]
            n139 = Strip Path(path=w736) -> (stripped path=w735:path)  [unwired: 1 out]
            n140 = Build Path(base path=w735, name or relative path=path "Antidoc-Output/Project-Documentation.adoc") -> (appended path=w734:path)
            n141 = call <vilib>:"Check if File or Folder Exists.vi"("path"=w734) -> ("file or folder exists?"=w732:bool, "dup path"=w733:path)  [unwired: 8 in, 1 out]
            n142 = case shown="False" w732 {
              tunnel: w733 -> [_ w743]
              frame False {
                n143 = invoke on="Generate Antidoc" class="Bool" method="ObjHighlight"() -> ()  [unwired: 3 in, 3 out]
                n144 = call "Status Updated.vi"("Status"="No Antidoc Output has been found, please\ngenerate it first") -> ()  [unwired: 10 in, 1 out]
              }
              frame True {
                n145 = call-poly <vilib>:"Open URL in Default Browser.vi"("path"=w743) -> ()  [unwired: 5 in, 2 out]
              }
            }
          }
          frame "Save Project Documentation" {
            n146 = Variant To Data(error in=w752, type=T28 {"Project Description"=""} ("Save Project Documentation Argument"), Variant=w749) -> (data=w747:T28, error out=w751:errorcluster)
            n147 = Unbundle By Name(w747) -> ("Project Description"=w744:string)
            n148 = Unbundle By Name(w746) -> ("DQMH Scan Results.Project References.Project Ref"=w745:refnum<vi>)
            n149 = property class="Project"(reference=w745, error in=w751, "Description"=w744) -> (error out=w750:errorcluster)  [unwired: 1 out]
          }
          frame "---Copy This Frame---" {
            # "Duplicate this frame when creating new messages.  Change this comment in the duplicated frame to describe this message."
            n150 = Merge Errors(w755) -> (w754:errorcluster)
          }
          frame "---Exit and Error Handling---" {
            # "Separator - The following cases handle errors and exit messages."
          }
          frame "Error" {
            # "Error - Check the error message data and respond accordingly. This message is sent by the \"Error Handler\" VIs at the end of each loop in this application."
            n151 = property on="Property Node" class="Module Admin"(reference=w759) -> ("Accessors:External Launch"=w758:bool)  [unwired: 1 in, 2 out]
            n152 = Variant To Data(error in=w767, type=errorcluster {"status"=FALSE, "code"=0, "source"=""} ("error constant"), Variant=w761) -> (data=w768:errorcluster, error out=w765:errorcluster)
            n153 = call "Error Reported.vi"("Error"=w768) -> ()  [unwired: 10 in, 1 out]
            n154 = case shown="True" w758 {
              tunnel: [w773 _] -> w764
              tunnel: w760 -> [w771 _]
              tunnel: w768 -> [w772 _]
              frame False {
                # "If the module is running standalone, then pop up an error dialog and call the \"Exit\" message."
                n155 = call <vilib>:"Simple Error Handler.vi"("error in (no error)"=w772) -> ()  [unwired: 4 in, 5 out]
                n156 = call-poly <vilib>:"Delacor_lib_QMH_Enqueue Message (poly).vi"("Priority Message? (F)"=TRUE, "Message"="Exit", "Message Queue in"=w771) -> ("error out"=w773:errorcluster)  [unwired: 7 in, 1 out]
              }
              frame True {
                # "If the module was launched externally, calling the Error Reported broadcast VI is the only action performed by the \"Error\" message. The module's caller can then process the error appropriately."
              }
            }
            n157 = Merge Errors(w765, w764) -> (w763:errorcluster)
            n158 = local write "error out"(w763) -> ()
          }
          frame "Exit" {
            w783 = 91  # 91: not all Exit messages will have an argument
            w785 = TRUE  # Stop the VI
            # "Store the last panel position"
            # "Release the message queue reference"
            # "Exit - Exit the application."
            n159 = Variant To Data(error in=w792, type=T20 {"Origin"="", "Exit via Stop Module Req?"=FALSE, "Wait for Module to stop?"=FALSE} ("Stop Argument"), Variant=w784) -> (data=w781:T20, error out=w788:errorcluster)
            n160 = call <vilib>:"Clear Errors.vi"("error in (no error)"=w788, "specific error code to clear (0: all)"=w783) -> ("error out"=w791:errorcluster)  [unwired: 4 in, 1 out]
            n161 = control-ref of="This VI"() -> (w780:refnum<vi>)
            n162 = invoke on="Modules Tree" class="Tree (strict)" method="Edit Tree Items.Delete"() -> ()  [unwired: 5 in, 5 out]
            n163 = call-dynamic "Delacor_lib_QMH_Release Message Queue.vi"("error in"=w791, "Message Queue"=w786) -> ("error out"=w790:errorcluster)  [unwired: 9 in]
            n164 = call "Handle Exit.vi"("Stop Argument"=w781, "Admin in"=w779, "VI reference"=w780) -> ("error out"=w787:errorcluster)  [unwired: 7 in, 1 out]
            n165 = call "Close vi references.vi"("Data Cluster"=w778) -> ()  [unwired: 10 in, 1 out]
            n166 = control-ref of="This VI"() -> (w777:refnum<vi>)
            n167 = Merge Errors(w790, w787) -> (w789:errorcluster)
            n168 = property class="VI"(reference=w777) -> ("Front Panel.PanelBounds"=w776:T30)  [unwired: 1 in, 2 out]
            n169 = call "Module Name--constant.vi"() -> ("Module Name"=w774:string)  [unwired: 11 in]
            n170 = call "Stop Module.vi"("Origin"="Panther Dahsboard Stopped") -> ()  [unwired: 10 in, 1 out]
            n171 = call "Save Window Position and Size.vi"("NewBnds"=w776, "Position Key"=w774) -> ()  [unwired: 9 in, 1 out]
          }
          frame Default {
            # "'Default' case only runs if there is a message that isn't defined in any of the other cases.  Output a programming error."
            n172 = call "Module Name--constant.vi"() -> ("Module Name"=w793:string)  [unwired: 11 in]
            n173 = xnode ("Error Ring")("parameter 0"=w794, "parameter 1"=w793) -> ("error out"=w798:errorcluster)
            n174 = Merge Errors(w796, w798) -> (w797:errorcluster)
          }
        }
        n175 = call-dynamic "Delacor_lib_QMH_Error Handler - Message Handling Loop.vi"("error in"=w467, "Ignore Errors (Runtime)"=w455, "Message Queue in"=w457) -> ("dup error in"=w464:errorcluster)  [unwired: 7 in, 1 out]
      }
      n176 = while {
        tunnel: w30 -> [w139]
        shift-right: [w141] -> w36
        shift-left: w34 -> [w142]
        tunnel: [w143] -> w39
        shift-right: [w137] -> _
        shift-left: w29 -> [w136]
        shift-right: [w135] -> _
        shift-left: Selection_Type--enum."Public API" ("Selection type") -> [w134]
        stop <- w140 stop-if-true
        # "Event Handling Loop"
        n177 = event "DQMH_EVENT_MAIN" shown="[36] <Panther Dashboard Request Events.Save Project Documentation>: User Event" {
          selector: w142 -> [_ _ _ _ _ _ _ _ _ _ _ _ _ _ _ _ _ _ _ _ _ _ _ _ _ _ _ _ _ _ _ _ _ _ _ _ _]
          dyn-events: [_ _ _ _ _ _ _ _ _ _ _ _ _ _ _ _ _ _ _ _ _ _ _ _ _ _ _ _ _ _ _ _ _ _ _ _ _] -> w141
          timeout: 3000 -> [_ _ _ _ _ _ _ _ _ _ _ _ _ _ _ _ _ _ _ _ _ _ _ _ _ _ _ _ _ _ _ _ _ _ _ _ _]
          tunnel: [_ _ _ _ _ _ _ _ _ _ _ _ _ _ _ _ _ _ _ _ TRUE ("Discard?") _ _ _ _ _ _ _ _ _ _ _ _ _ _ _ _] -> w140
          tunnel: w139 -> [_ w153 _ _ w188 w193 w205 w210 w235 _ w244 _ w258 w268 _ _ w285 w294 _ _ w327 w336 _ w347 w355 w363 w371 w379 w387 w395 w403 w411 w419 w427 w435 w443 w451]
          tunnel: [w149 w162 w176 w181 w189 w194 w206 w211 w236 w241 w247 w255 w261 w269 w273 _ w286 w295 _ _ w330 w338 w342 w350 w358 w366 w374 w382 w390 w398 w406 w414 w422 w430 w438 w446 w454] -> w144
          tunnel: [w148 w161 w175 w180 w183 w191 w202 w208 w231 w237 w246 w254 w260 w263 w271 w275 w279 w292 w307 w318 w320 w333 w341 w349 w357 w365 w373 w381 w389 w397 w405 w413 w421 w429 w437 w445 w453] -> w137
          tunnel: w136 -> [w148 w161 w175 w180 w183 w191 w202 w208 _ w237 w246 w254 w260 w263 w271 w275 w279 w292 w307 w318 w320 w333 w341 w349 w357 w365 w373 w381 w389 w397 w405 w413 w421 w429 w437 w445 w453]
          tunnel: [w147 w160 w174 w179 w182 w190 w201 w207 w229 w239 w245 w253 w259 w262 w270 w274 w278 w291 w306 w317 w319 w332 w340 w348 w356 w364 w372 w380 w388 w396 w404 w412 w420 w428 w436 w444 w452] -> w135
          tunnel: w134 -> [w147 w160 w174 w179 w182 _ w201 w207 _ w239 w245 w253 w259 w262 w270 w274 w278 w291 w306 w317 w319 w332 w340 w348 w356 w364 w372 w380 w388 w396 w404 w412 w420 w428 w436 w444 w452]
          event Panel Resize {
            n178 = event-data() -> ("NewBnds"=w145:T30)  [unwired: 1 in]
            n179 = First Call?() -> (First Call?: T/F=w146:bool)
            n180 = case shown="False" w146 {
              tunnel: [w152 _] -> w149
              tunnel: w145 -> [w151 _]
              frame False {
                n181 = call "Module Name--constant.vi"() -> ("Module Name"=w150:string)  [unwired: 11 in]
                n182 = call "Save Window Position and Size.vi"("NewBnds"=w151, "Position Key"=w150) -> ("error out"=w152:errorcluster)  [unwired: 9 in]
              }
              frame True {
              }
            }
          }
          event "Add Event", "Remove Event", "Convert Event", "Rename Event", "Add New Module", "Rename Module", "Validate Module", "Create Module Template", "Add Unit Test Module", "Create RT Tester Module": Value Change {
            n183 = event-data() -> ("CtlRef"=w158:refnum<vi>)  [unwired: 1 in]
            n184 = property class="Bool"(reference=w158) -> ("Label.Text"=w159:string)  [unwired: 1 in, 2 out]
            n185 = case shown="\"Create Module Template\"" w159 {
              tunnel: [DQMH_Tools_Menu--enum."Create New DQMH Event" ("DQMH Tools") DQMH_Tools_Menu--enum."Convert DQMH Event" ("DQMH Tools") DQMH_Tools_Menu--enum."Remove DQMH Event" ("DQMH Tools") DQMH_Tools_Menu--enum."Rename DQMH Event" ("DQMH Tools") DQMH_Tools_Menu--enum."Add New DQMH Module" ("DQMH Tools") DQMH_Tools_Menu--enum."Rename DQMH Module" ("DQMH Tools") DQMH_Tools_Menu--enum."Validate DQMH Module" ("DQMH Tools") DQMH_Tools_Menu--enum."Create RT Tester" ("DQMH Tools") DQMH_Tools_Menu--enum."New DQMH  Unit Test" ("DQMH Tools") DQMH_Tools_Menu--enum."Create DQMH Module Template" ("DQMH Tools")] -> w154
              frame "Add Event", Default {
              }
              frame "Convert Event" {
              }
              frame "Remove Event" {
              }
              frame "Rename Event" {
              }
              frame "Add New Module" {
              }
              frame "Rename Module" {
              }
              frame "Validate Module" {
              }
              frame "Create RT Tester Module" {
              }
              frame "Add Unit Test Module" {
              }
              frame "Create Module Template" {
              }
            }
            n186 = Bundle(cluster=T13 {"Scripting Tool"=enum."Create New DQMH Event"} ("Launch DQMH Scripting Tools Argument"), "Scripting Tool"=w154) -> (w157:T13)
            n187 = call-poly <vilib>:"Delacor_lib_QMH_Enqueue Message (poly).vi"("Message Data"=w157, "Message"="Launch DQMH Scripting Tools", "Message Queue in"=w153) -> ("error out"=w162:errorcluster)  [unwired: 7 in, 1 out]
          }
          event "Doc Editor": Value Change {
            # "Open Documentation DQMH Module"
            n188 = event-data() -> ()  [unwired: 1 in, 1 out]
            n189 = case shown="True" "Doc Editor" {
              tunnel: [w177 w178] -> w176
              frame False {
                n190 = call "Hide Panel.vi"() -> ("error out"=w177:errorcluster)  [unwired: 11 in]
              }
              frame True {
                n191 = call "Show Panel.vi"() -> ("error out"=w178:errorcluster)  [unwired: 11 in]
              }
            }
          }
          event User Event {
            # "We wait for the Context help module to init to request to refresh \npanther Dashboard Broadcasts, we need this module to be\nlistening Panther Dashboard broadcasts"
            n192 = event-data() -> ()  [unwired: 1 in, 1 out]
            n193 = call "Refresh Panther Dashboard Broadcasts.vi"() -> ("error out"=w181:errorcluster)  [unwired: 11 in]
          }
          event "Expand Results": Value Change {
            # "Expand or close Result tree"
            n194 = event-data() -> ()  [unwired: 1 in, 1 out]
            n195 = Bundle(cluster=T15 {"Expand?"=FALSE} ("Expand or Close Argument"), "Expand?"="Expand Results") -> (w185:T15)
            n196 = call-poly <vilib>:"Delacor_lib_QMH_Enqueue Message (poly).vi"("Message Data"=w185, "Message"="Expand or Close", "Message Queue in"=w188) -> ("error out"=w189:errorcluster)  [unwired: 7 in, 1 out]
          }
          event "Modules Tree": Double Click {
            # "User double click an element on the tree control, we check if it is an event to find its frame on the corresponding DQMH module, we also check if it is a broadcast to find where is being triggered"
            n197 = event-data() -> ("Tag"=w192:string)  [unwired: 1 in]
            n198 = call "Validate if event is selected.vi"("Tree Selection"=w192) -> ("Selection type"=w190:T4)  [unwired: 10 in]
            n199 = case shown="\"Module\"" w190 {
              tunnel: [w197 _ w200] -> w194
              tunnel: w193 -> [w196 _ w199]
              frame "Module" {
                # "Selection is a module"
                n200 = call-poly <vilib>:"Delacor_lib_QMH_Enqueue Message (poly).vi"("Message"="Find Module in project", "Message Queue in"=w196) -> ("error out"=w197:errorcluster)  [unwired: 8 in, 1 out]
              }
              frame "Public API" {
              }
              frame "Broadcast", "Request" {
                # "Selection is an Event vi?"
                n201 = call-poly <vilib>:"Delacor_lib_QMH_Enqueue Message (poly).vi"("Message"="Locate Event on Main", "Message Queue in"=w199) -> ("error out"=w200:errorcluster)  [unwired: 8 in, 1 out]
              }
            }
          }
          event "Modules Tree": Drag Starting? {
            # "Drag current selection to user destination"
            n202 = event-data() -> ()  [unwired: 1 in, 1 out]
            n203 = call-poly <vilib>:"Delacor_lib_QMH_Enqueue Message (poly).vi"("Message"="Drag VI", "Message Queue in"=w205) -> ("error out"=w206:errorcluster)  [unwired: 8 in, 1 out]
            n204 = event-data("Discard?"=TRUE) -> ()  [unwired: 1 in, 1 out]
          }
          event "Modules Tree": Shortcut Menu Selection (User) {
            # "User selects something from the Right Click Shortcut Menu"
            n205 = event-data() -> ("ItemTag"=w209:string)  [unwired: 1 in]
            n206 = case shown="\"Open File Library on Disk\", \"Open VI on Disk\", \"Who is launching this module?\"" w209 {
              selector: w209 -> [w214 _ w220 w223 w226]
              tunnel: w210 -> [w218 _ w221 w224 w227]
              tunnel: [w219 _ w222 w225 w228] -> w211
              frame "-Run: Hide Panel", "-Run: Show Diagram", "-Run: Show Panel", "-Run: Stop Module" {
                n207 = Match Pattern(string=w214, regular expression="-Run: ") -> (after substring=w213:string)  [unwired: 1 in, 3 out]
                n208 = Bundle(cluster=T16 {"Event Name"=""} ("Execute Default Event Request Argument"), "Event Name"=w213) -> (w216:T16)
                n209 = call-poly <vilib>:"Delacor_lib_QMH_Enqueue Message (poly).vi"("Message Data"=w216, "Message"="Execute Default Event Request", "Message Queue in"=w218) -> ("error out"=w219:errorcluster)  [unwired: 7 in, 1 out]
              }
              frame Default {
              }
              frame "Open File Library on Disk", "Open VI on Disk", "Who is launching this module?" {
                n210 = call-poly <vilib>:"Delacor_lib_QMH_Enqueue Message (poly).vi"("Message"=w220, "Message Queue in"=w221) -> ("error out"=w222:errorcluster)  [unwired: 8 in, 1 out]
              }
              frame "Who is registered to this module's broadcasts?" {
                n211 = call-poly <vilib>:"Delacor_lib_QMH_Enqueue Message (poly).vi"("Message"=w223, "Message Queue in"=w224) -> ("error out"=w225:errorcluster)  [unwired: 8 in, 1 out]
              }
              frame "Open Module API Tester", "Search for Event Callers / listeners" {
                n212 = call-poly <vilib>:"Delacor_lib_QMH_Enqueue Message (poly).vi"("Message"=w226, "Message Queue in"=w227) -> ("error out"=w228:errorcluster)  [unwired: 8 in, 1 out]
              }
            }
          }
          event "Modules Tree": Value Change {
            w231 = TRUE  # Tree valid Selection
            # "The user selected an item on the tree control"
            n213 = event-data() -> ()  [unwired: 1 in, 1 out]
            n214 = Bundle(cluster=T17 {"Tree DQMH Sel"=""} ("Tree DQMH Selection Argument"), "Tree DQMH Sel"="Modules Tree") -> (w232:T17)
            n215 = call "Validate if event is selected.vi"("Tree Selection"="Modules Tree") -> ("Selection type"=w229:T4)  [unwired: 10 in]
            n216 = call-poly <vilib>:"Delacor_lib_QMH_Enqueue Message (poly).vi"("Message Data"=w232, "Message"="Tree DQMH Selection", "Message Queue in"=w235) -> ("error out"=w236:errorcluster)  [unwired: 7 in, 1 out]
          }
          event "Modules Tree": Shortcut Menu Activation? {
            # "This is wher the shorcut menu is filled, only after the user select a module"
            n217 = event-data() -> ("MenuRef"=w240:refnum<k9>)  [unwired: 1 in]
            n218 = call "Create Tree Shortcut Menu.vi"("Selection type"=w239, "Menu in"=w240) -> ("error out"=w241:errorcluster)  [unwired: 9 in]
            n219 = Not(x=w237) -> (.not. x?=w238:bool)
            n220 = event-data("Discard?"=w238) -> ()  [unwired: 1 in, 1 out]
          }
          event "Projects": Value Change {
            n221 = event-data() -> ()  [unwired: 1 in, 1 out]
            n222 = call-poly <vilib>:"Delacor_lib_QMH_Enqueue Message (poly).vi"("Message Data"="Projects", "Message"="Refresh Targets", "Message Queue in"=w244) -> ("error out"=w247:errorcluster)  [unwired: 7 in, 1 out]
          }
          event "Projects": Shortcut Menu Activation? {
            n223 = event-data() -> ("MenuRef"=w252:refnum<k9>)  [unwired: 1 in]
            n224 = Delete Menu Items(9:w252) -> (0:w256:errorcluster, 3:w251:refnum<k9>)  [unwired: 3 in]
            n225 = Insert Menu Items(6:w256, 8:string[] ["Open Project Folder"] ("item names"), 9:w251) -> (0:w255:errorcluster)  [unwired: 3 in, 2 out]
            n226 = local read "Projects"() -> (w249:string)
            n227 = Empty String/Path?(string/path=w249) -> (empty?=w248:bool)
            n228 = event-data("Discard?"=w248) -> ()  [unwired: 1 in, 1 out]
          }
          event "Projects": Shortcut Menu Selection (User) {
            n229 = event-data() -> ("ItemTag"=w257:string)  [unwired: 1 in]
            n230 = call-poly <vilib>:"Delacor_lib_QMH_Enqueue Message (poly).vi"("Message"=w257, "Message Queue in"=w258) -> ("error out"=w261:errorcluster)  [unwired: 8 in, 1 out]
          }
          event User Event {
            # "Another Module called the \"Expand or Close\" API Method."
            n231 = event-data() -> ("Expand?"=w264:bool)  [unwired: 1 in]
            n232 = Bundle(cluster=T15 {"Expand?"=FALSE} ("Expand or Close Argument"), "Expand?"=w264) -> (w265:T15)
            n233 = call-poly <vilib>:"Delacor_lib_QMH_Enqueue Message (poly).vi"("Message Data"=w265, "Message"="Expand or Close", "Message Queue in"=w268) -> ("error out"=w269:errorcluster)  [unwired: 7 in, 1 out]
          }
          event User Event {
            # "Another Module called the \"Get Module Execution Status\" API Method."
            n234 = event-data() -> ()  [unwired: 1 in, 1 out]
            n235 = call "Update Module Execution Status.vi"("Running?"=TRUE) -> ("error out"=w273:errorcluster)  [unwired: 10 in]
          }
          event User Event {
            # "Hide the panel of this VI, and send a status updated message to let listeners know."
            # "Another Module called the \"Hide Panel\" API Method."
            n236 = event-data() -> ()  [unwired: 1 in, 1 out]
            n237 = control-ref of="This VI"() -> (w276:refnum<vi>)
            n238 = call "Hide VI Panel.vi"("VI"=w276) -> ()  [unwired: 10 in, 1 out]
          }
          event User Event {
            # "Another Module called the \"Scan DQMH Modules\" API Method."
            n239 = event-data() -> ("Include Dependencies"=w281:bool, "Project"=w280:string, "Target"=w277:string)  [unwired: 1 in]
            n240 = Bundle(cluster=T18 {"Include Dependencies"=FALSE, "Project"="", "Target"=""} ("Scan DQMH Modules Argument"), "Include Dependencies"=w281, "Project"=w280, "Target"=w277) -> (w282:T18)
            n241 = call-poly <vilib>:"Delacor_lib_QMH_Enqueue Message (poly).vi"("Message Data"=w282, "Message"="Scan DQMH Modules", "Message Queue in"=w285) -> ("error out"=w286:errorcluster)  [unwired: 7 in, 1 out]
          }
          event "Search": Value Change {
            # "#via_ignore Unwired Event Nodes"
            # "Another Module called the \"Scan DQMH Modules\" API Method."
            n242 = event-data() -> ()  [unwired: 1 in, 1 out]
            n243 = local read "Projects"() -> (w290:string)
            n244 = Empty String/Path?(string/path="Targets") -> (empty?=w288:bool)
            n245 = global write "Panther Dashboard--global.vi" "Target"("Targets") -> ()
            n246 = Empty String/Path?(string/path=w290) -> (empty?=w293:bool)
            n247 = Or(x=w293, y=w288) -> (x .or. y?=w289:bool)
            n248 = case shown="True" w289 {
              tunnel: [w303 _] -> w295
              tunnel: w294 -> [w302 _]
              tunnel: w290 -> [w297 _]
              tunnel: "Targets" -> [w296 _]
              frame False {
                n249 = Bundle(cluster=T18 {"Include Dependencies"=FALSE, "Project"="", "Target"=""} ("Scan DQMH Modules Argument"), "Include Dependencies"="Include Dependencies", "Project"=w297, "Target"=w296) -> (w299:T18)
                n250 = call-poly <vilib>:"Delacor_lib_QMH_Enqueue Message (poly).vi"("Message Data"=w299, "Message"="Scan DQMH Modules", "Message Queue in"=w302) -> ("error out"=w303:errorcluster)  [unwired: 7 in, 1 out]
              }
              frame True {
                n251 = invoke on="Projects" class="CmbBox" method="ObjHighlight"() -> (error out=w305:errorcluster)  [unwired: 3 in, 2 out]
                n252 = invoke on="Targets" class="CmbBox" method="ObjHighlight"(error in=w305) -> ()  [unwired: 2 in, 3 out]
                n253 = call "Status Updated.vi"("Status"="Scanning requires a project and an target please make the selection.\n") -> ()  [unwired: 10 in, 1 out]
              }
            }
          }
          event User Event {
            # "Another Module called the \"Show Diagram\" API Method. This event is used for debugging."
            n254 = event-data() -> ()  [unwired: 1 in, 1 out]
            n255 = disable-structure shown="RUN_TIME_ENGINE==False" {
              frame condition #0 (active) {
                # "functionality not available in exe"
                n256 = invoke on="Invoke Node" class="VI" method="Lock State.Get"() -> (error out=w313:errorcluster, "Get Lock State"=w312:T19, "pwd in cache"=w309:bool)  [unwired: 4 in, 1 out]
                n257 = Equal?(x=T19."Password-protected", y=w312) -> (x = y?=w310:bool)
                n258 = Compound Arithmetic op=AND(w310, invert w309) -> (w308:bool)
                n259 = case shown="False" w308 {
                  tunnel: w313 -> [w315 _]
                  frame False {
                    n260 = property on="Property Node" class="VI"(error in=w315, "BDWin.Open"=TRUE ("Block Diagram Window:Open")) -> ()  [unwired: 1 in, 2 out]
                  }
                  frame True {
                    # "Password-protected VI, and the password is not in the cache. Do not show the diagram."
                  }
                }
              }
              frame condition #1 {
              }
            }
          }
          event User Event {
            # "Show the panel of this VI, and send a status updated message to let listeners know."
            # "Another Module called the \"Show Panel\" API Method."
            n261 = event-data() -> ()  [unwired: 1 in, 1 out]
            n262 = control-ref of="This VI"() -> (w316:refnum<vi>)
            n263 = call "Open VI Panel.vi"("VI"=w316) -> ()  [unwired: 10 in, 1 out]
          }
          event User Event {
            # "The Stop Module Event can get fired from the Exit message in the MHL. The queue gets destroyed in that case. If the queue no longer exists, the Enqueue Exit as a priority message will return error 1. It is safe to ignore, because the module is already exiting."
            # "Another Module called the \"Stop Module\" API Method  or the Message Handling Loop below."
            n264 = event-data() -> ("Exit via Stop Module Req?"=w323:bool, "Wait for Module to stop?"=w322:bool)  [unwired: 1 in]
            n265 = Bundle By Name(cluster=T20 {"Origin"="", "Exit via Stop Module Req?"=FALSE, "Wait for Module to stop?"=FALSE} ("Stop Argument"), "Exit via Stop Module Req?"=w323, "Wait for Module to stop?"=w322) -> (w321:T20)
            n266 = call-poly <vilib>:"Delacor_lib_QMH_Enqueue Message (poly).vi"("Priority Message? (F)"=TRUE, "Message Data"=w321, "Message"="Exit", "Message Queue in"=w327) -> ("error out"=w331:errorcluster)  [unwired: 6 in, 1 out]
            n267 = call <vilib>:"Clear Errors.vi"("error in (no error)"=w331, "specific error code to clear (0: all)"=1) -> ("error out"=w330:errorcluster)  [unwired: 4 in, 1 out]
          }
          event Panel Close? {
            w337 = TRUE  # Discard the event, the MHL is responsible for closing and stopping this VI.
            # "Hide the panel or send the 'Exit' message if the user clicks the 'X' on the module main VI panel."
            n268 = event-data() -> ()  [unwired: 1 in, 1 out]
            n269 = call-poly <vilib>:"Delacor_lib_QMH_Enqueue Message (poly).vi"("Priority Message? (F)"=TRUE, "Message"="Exit", "Message Queue in"=w336) -> ("error out"=w338:errorcluster)  [unwired: 7 in, 1 out]
            n270 = event-data ("Event Filter Node")("Discard?"=w337) -> ()  [unwired: 1 in, 1 out]
          }
          event Timeout {
            n271 = event-data() -> ()  [unwired: 1 in, 1 out]
            n272 = call "Scan For App Projects.vi"("Init?"=FALSE) -> ("error out"=w342:errorcluster)  [unwired: 10 in]
          }
          event User Event {
            # "Another Module called the \"Launch DQMH Scripting Tools\" API Method."
            n273 = event-data() -> ("Scripting Tool"=w343:T14)  [unwired: 1 in]
            n274 = Bundle(cluster=T13 {"Scripting Tool"=enum."Create New DQMH Event"} ("Launch DQMH Scripting Tools Argument"), "Scripting Tool"=w343) -> (w344:T13)
            n275 = call-poly <vilib>:"Delacor_lib_QMH_Enqueue Message (poly).vi"("Message Data"=w344, "Message"="Launch DQMH Scripting Tools", "Message Queue in"=w347) -> ("error out"=w350:errorcluster)  [unwired: 7 in, 1 out]
          }
          event User Event {
            # "Another Module called the \"Generate Project Documentation\" API Method."
            n276 = event-data() -> ("Boolean"=w351:bool)  [unwired: 1 in]
            n277 = Bundle(cluster=T21 {"Boolean"=FALSE} ("Generate Project Documentation Argument"), "Boolean"=w351) -> (w352:T21)
            n278 = call-poly <vilib>:"Delacor_lib_QMH_Enqueue Message (poly).vi"("Message Data"=w352, "Message"="Generate Project Documentation", "Message Queue in"=w355) -> ("error out"=w358:errorcluster)  [unwired: 7 in, 1 out]
          }
          event "Generate Antidoc": Value Change {
            # "Another Module called the \"Generate Project Documentation\" API Method."
            n279 = event-data() -> ()  [unwired: 1 in, 1 out]
            n280 = Bundle(cluster=T21 {"Boolean"=FALSE} ("Generate Project Documentation Argument"), "Boolean"="Generate Antidoc") -> (w360:T21)
            n281 = call-poly <vilib>:"Delacor_lib_QMH_Enqueue Message (poly).vi"("Message Data"=w360, "Message"="Generate Project Documentation", "Message Queue in"=w363) -> ("error out"=w366:errorcluster)  [unwired: 7 in, 1 out]
          }
          event User Event {
            # "Another Module called the \"Set App Theme\" API Method."
            n282 = event-data() -> ("Theme"=w367:bool)  [unwired: 1 in]
            n283 = Bundle(cluster=T22 {"Theme"=FALSE} ("Set App Theme Argument"), "Theme"=w367) -> (w368:T22)
            n284 = call-poly <vilib>:"Delacor_lib_QMH_Enqueue Message (poly).vi"("Message Data"=w368, "Message"="Set App Theme", "Message Queue in"=w371) -> ("error out"=w374:errorcluster)  [unwired: 7 in, 1 out]
          }
          event "Theme Panther": Value Change {
            # "Another Module called the \"Set App Theme\" API Method."
            n285 = event-data() -> ()  [unwired: 1 in, 1 out]
            n286 = Bundle(cluster=T22 {"Theme"=FALSE} ("Set App Theme Argument"), "Theme"="Theme Panther") -> (w376:T22)
            n287 = call-poly <vilib>:"Delacor_lib_QMH_Enqueue Message (poly).vi"("Message Data"=w376, "Message"="Set App Theme", "Message Queue in"=w379) -> ("error out"=w382:errorcluster)  [unwired: 7 in, 1 out]
          }
          event User Event {
            # "Another Module called the \"Show About\" API Method."
            n288 = event-data() -> ("Boolean"=w383:bool)  [unwired: 1 in]
            n289 = Bundle(cluster=T23 {"Boolean"=FALSE} ("Show About Argument"), "Boolean"=w383) -> (w384:T23)
            n290 = call-poly <vilib>:"Delacor_lib_QMH_Enqueue Message (poly).vi"("Message Data"=w384, "Message"="Show About", "Message Queue in"=w387) -> ("error out"=w390:errorcluster)  [unwired: 7 in, 1 out]
          }
          event "About Panther": Value Change {
            # "Another Module called the \"Show About\" API Method."
            n291 = event-data() -> ()  [unwired: 1 in, 1 out]
            n292 = Bundle(cluster=T23 {"Boolean"=FALSE} ("Show About Argument"), "Boolean"="About Panther") -> (w392:T23)
            n293 = call-poly <vilib>:"Delacor_lib_QMH_Enqueue Message (poly).vi"("Message Data"=w392, "Message"="Show About", "Message Queue in"=w395) -> ("error out"=w398:errorcluster)  [unwired: 7 in, 1 out]
          }
          event User Event {
            # "Another Module called the \"Update Module ID\" API Method."
            n294 = event-data() -> ("New ID"=w399:i32)  [unwired: 1 in]
            n295 = Bundle(cluster=T24 {"New ID"=-1} ("Update Module ID Argument"), "New ID"=w399) -> (w400:T24)
            n296 = call-poly <vilib>:"Delacor_lib_QMH_Enqueue Message (poly).vi"("Message Data"=w400, "Message"="Update Module ID", "Message Queue in"=w403) -> ("error out"=w406:errorcluster)  [unwired: 7 in, 1 out]
          }
          event "Module ID": Value Change {
            # "Another Module called the \"Update Module ID\" API Method."
            n297 = event-data() -> ()  [unwired: 1 in, 1 out]
            n298 = Bundle(cluster=T24 {"New ID"=-1} ("Update Module ID Argument"), "New ID"="Module ID") -> (w408:T24)
            n299 = call-poly <vilib>:"Delacor_lib_QMH_Enqueue Message (poly).vi"("Message Data"=w408, "Message"="Update Module ID", "Message Queue in"=w411) -> ("error out"=w414:errorcluster)  [unwired: 7 in, 1 out]
          }
          event User Event {
            # "Another Module called the \"Save Library Description\" API Method."
            n300 = event-data() -> ("Library Description"=w415:string)  [unwired: 1 in]
            n301 = Bundle(cluster=T25 {"Library Description"=""} ("Save Library Description Argument"), "Library Description"=w415) -> (w416:T25)
            n302 = call-poly <vilib>:"Delacor_lib_QMH_Enqueue Message (poly).vi"("Message Data"=w416, "Message"="Save Library Description", "Message Queue in"=w419) -> ("error out"=w422:errorcluster)  [unwired: 7 in, 1 out]
          }
          event User Event {
            # "Another Module called the \"Save VI Description\" API Method."
            n303 = event-data() -> ("VI Description"=w423:string)  [unwired: 1 in]
            n304 = Bundle(cluster=T26 {"VI Description"=""} ("Save VI Description Argument"), "VI Description"=w423) -> (w424:T26)
            n305 = call-poly <vilib>:"Delacor_lib_QMH_Enqueue Message (poly).vi"("Message Data"=w424, "Message"="Save VI Description", "Message Queue in"=w427) -> ("error out"=w430:errorcluster)  [unwired: 7 in, 1 out]
          }
          event User Event {
            # "Another Module called the \"Open Documentation\" API Method."
            n306 = event-data() -> ("Boolean"=w431:bool)  [unwired: 1 in]
            n307 = Bundle(cluster=T27 {"Boolean"=FALSE} ("Open Documentation Argument"), "Boolean"=w431) -> (w432:T27)
            n308 = call-poly <vilib>:"Delacor_lib_QMH_Enqueue Message (poly).vi"("Message Data"=w432, "Message"="Open Documentation", "Message Queue in"=w435) -> ("error out"=w438:errorcluster)  [unwired: 7 in, 1 out]
          }
          event "Open Antidoc Output": Value Change {
            # "Another Module called the \"Open Documentation\" API Method."
            n309 = event-data() -> ()  [unwired: 1 in, 1 out]
            n310 = Bundle(cluster=T27 {"Boolean"=FALSE} ("Open Documentation Argument"), "Boolean"="Open Antidoc Output") -> (w440:T27)
            n311 = call-poly <vilib>:"Delacor_lib_QMH_Enqueue Message (poly).vi"("Message Data"=w440, "Message"="Open Documentation", "Message Queue in"=w443) -> ("error out"=w446:errorcluster)  [unwired: 7 in, 1 out]
          }
          event User Event {
            # "Another Module called the \"Save Project Documentation\" API Method."
            n312 = event-data() -> ("Project Description"=w447:string)  [unwired: 1 in]
            n313 = Bundle(cluster=T28 {"Project Description"=""} ("Save Project Documentation Argument"), "Project Description"=w447) -> (w448:T28)
            n314 = call-poly <vilib>:"Delacor_lib_QMH_Enqueue Message (poly).vi"("Message Data"=w448, "Message"="Save Project Documentation", "Message Queue in"=w451) -> ("error out"=w454:errorcluster)  [unwired: 7 in, 1 out]
          }
        }
        n315 = call-dynamic "Delacor_lib_QMH_Error Handler - Event Handling Loop.vi"("error in"=w144, "Message Queue in"=w139) -> ("dup error in"=w143:errorcluster)  [unwired: 8 in, 1 out]
      }
      n316 = while {
        tunnel: w33 -> [w50]
        tunnel: [w49] -> w32
        shift-right: [w47] -> _
        shift-left: -1 -> [w46]
        shift-right: [w45] -> _
        shift-left: _ -> [w44]
        tunnel: w30 -> [w43]
        tunnel: [w51] -> w37
        shift-right: [w42] -> _
        shift-left: _ -> [w41]
        stop <- w48 stop-if-true
        # "Helper Loop"
        n317 = event shown="[7] <Panther Dashboard Request Events.Register controls Mouse Enter>: User Event" {
          selector: w50 -> [_ _ _ _ _ _ _ w111 _ _ _]
          dyn-events: [_ _ _ _ _ _ _ w109 _ _ _] -> w49
          timeout: w46 -> [_ _ _ _ _ _ _ _ _ _ _]
          tunnel: [_ TRUE _ _ _ _ _ _ _ _ _] -> w48
          tunnel: [w54 w59 w64 w77 w88 w92 w104 w110 w118 w129 w133] -> w45
          tunnel: [w55 w60 500 w76 w87 w91 w103 w113 w117 w128 w132] -> w47
          tunnel: w46 -> [w55 w60 _ w76 w87 w91 w103 w113 w117 w128 w132]
          tunnel: w44 -> [w54 w59 _ w77 w88 w92 w104 w110 w118 w129 w133]
          tunnel: [w56 _ _ _ _ _ _ _ w119 _ _] -> w52
          tunnel: [w53 w57 w62 w75 w85 w90 w102 w112 w116 w127 w131] -> w42
          tunnel: w41 -> [w53 w57 _ w75 w85 w90 w102 w112 w116 w127 w131]
          event Timeout {
            n318 = event-data() -> ()  [unwired: 1 in, 1 out]
            n319 = call "Get Module Execution Status by ref.vi"("Modules Tree ref"=w53, "Refs"=w54) -> ("error out"=w56:errorcluster)  [unwired: 9 in]
          }
          event User Event {
            n320 = event-data() -> ()  [unwired: 1 in, 1 out]
            n321 = Unbundle By Name(w59) -> ("Modules"=w58:refnum<vi>[])
            n322 = Close Reference(reference=w58) -> ()  [unwired: 1 in, 1 out]
          }
          event User Event {
            # "Refresh time"
            n323 = event-data() -> ("Modules"=w67:refnum<vi>[], "Modules Types"=w65:T9[], "Application Instance"=w66:refnum<vi>)  [unwired: 1 in]
            n324 = Bundle By Name(cluster=T11 {"Modules"=[], "Modules Types"=[], "Application Instance"=refnum}, "Modules"=w67, "Modules Types"=w65, "Application Instance"=w66) -> (w64:T11)
            n325 = control-ref of="Modules Tree"() -> (w63:refnum<vi>)
            n326 = call "Set Tree custom symbols.vi"("TreeControl in"=w63) -> ("TreeControl out"=w62:refnum<vi>)  [unwired: 10 in]
          }
          event User Event {
            n327 = event-data() -> ("Projects"=w73:string[])  [unwired: 1 in]
            n328 = Array Size(array=w73) -> (size(s)=w72:i32)
            n329 = Equal?(x=1, y=w72) -> (x = y?=w70:bool)
            n330 = control-ref of="Projects"() -> (w74:refnum<vi>)
            n331 = case shown="True" w70 {
              tunnel: w74 -> [w80 w82]
              tunnel: w73 -> [w79 w81]
              frame True {
                n332 = Index Array(array=w79) -> (element=w78:string)  [unwired: 1 in]
                n333 = property class="CmbBox"(reference=w80, "Strings[]"=w79, "Val(Sgnl)"=w78) -> ()  [unwired: 1 in, 2 out]
              }
              frame False {
                n334 = property class="CmbBox"(reference=w82, "Strings[]"=w81) -> ()  [unwired: 1 in, 2 out]
              }
            }
          }
          event User Event {
            n335 = event-data() -> ("Targets"=w84:string[])  [unwired: 1 in]
            n336 = Index Array(array=w84) -> (element=w83:string)  [unwired: 1 in]
            n337 = control-ref of="Targets"() -> (w86:refnum<vi>)
            n338 = property class="CmbBox"(reference=w86, "Strings[]"=w84, "Value"=w83) -> ()  [unwired: 1 in, 2 out]
          }
          event User Event {
            n339 = event-data() -> ("Progress"=→"Progress":u16)  [unwired: 1 in]
          }
          event Mouse Enter {
            n340 = event-data() -> ("CtlRef"=w93:refnum<vi>)  [unwired: 1 in]
            n341 = property class="Ctl"(reference=w93) -> ("Label.Text"=w99:string, "TipStrip"=w100:string)  [unwired: 1 in, 2 out]
            n342 = control-ref of="antidoc"() -> (w94:refnum<vi>)
            n343 = control-ref of="Panther Indicator"() -> (w98:refnum<vi>)
            n344 = control-ref of="Process Indicator"() -> (w97:refnum<vi>)
            n345 = control-ref of="Event Indicator"() -> (w96:refnum<vi>)
            n346 = Empty String/Path?(string/path=w100) -> (empty?=w101:bool)
            n347 = Build Array(w94, w98, w97, w96) -> (w95:refnum<vi>[])
            n348 = call "Set Indicators Visibility Status.vi"("Indicator Refs"=w95, "Label"=w99) -> ()  [unwired: 10 in]
            n349 = case shown="False" w101 {
              tunnel: w100 -> [w105 _]
              frame False {
                n350 = call "Status Updated.vi"("Status"=w105) -> ()  [unwired: 10 in, 1 out]
              }
              frame True {
              }
            }
          }
          event User Event {
            n351 = event-data() -> ()  [unwired: 1 in, 1 out]
            n352 = control-ref of="This VI"() -> (w107:refnum<vi>)
            n353 = property class="VI"(reference=w107) -> ("Panel"=w108:refnum<vi>)  [unwired: 1 in, 2 out]
            n354 = property class="Pnl"(reference=w108) -> ("Controls[]"=w106:refnum<vi>[])  [unwired: 1 in, 2 out]
            n355 = register-events(reference=w111, w106) -> (reference out=w109:refnum<event-registration>)  [unwired: 3 in, 1 out]
          }
          event User Event {
            n356 = event-data() -> ("Scale Max"=w115:i32)  [unwired: 1 in]
            n357 = control-ref of="Progress"() -> (w114:refnum<vi>)
            n358 = property class="Slide (strict)"(reference=w114, "Scale.Maximum"=w115) -> (error out=w119:errorcluster)  [unwired: 1 in, 1 out]
          }
          event User Event {
            n359 = event-data() -> ("Module Type"=w126:T9)  [unwired: 1 in]
            n360 = Equal?(x=Module_type--enum."Module type: Cloneable", y=w126) -> (x = y?=w124:bool)
            n361 = Select(t=T12."Enabled" ("Disabled"), s=w124, f=T12."Disabled and Grayed Out") -> (s? t:f=w121:T12)
            n362 = control-ref of="Module ID"() -> (w123:refnum<vi>)
            n363 = property class="DigNum (strict)"(reference=w123, "DisabledEnum"=w121) -> ()  [unwired: 1 in, 2 out]
          }
          event User Event {
            n364 = event-data() -> ("Status"=→"Status":string)  [unwired: 1 in]
          }
        }
        n365 = call-dynamic "Delacor_lib_QMH_Error Handler - Helper Loop.vi"("error in"=w52, "Message Queue in"=w43) -> ("dup error in"=w51:errorcluster)  [unwired: 8 in, 1 out]
      }
    }
    frame Error {
      # "Synchronize Caller Events.vi will inform Start Module.vi that the module has launched and will let the code calling Start Module.vi register for broadcasts and would permit the caller receive the broadcast that an error occurred at launch time."
      n366 = call-dynamic "Delacor_lib_QMH_Release Message Queue.vi"("error in"=w815, "Message Queue"=w809) -> ("error out"=w814:errorcluster)  [unwired: 9 in]
      n367 = call "Synchronize Caller Events.vi"("Singleton Module Admin in"=w810) -> ("error out"=w816:errorcluster)  [unwired: 9 in, 1 out]
      n368 = call "Module Name--constant.vi"() -> ("Module Name"=w812:string)  [unwired: 11 in]
      n369 = Format Into String(format string="An error occurred during initialization. %s is no longer running.", w812) -> (resulting string=w807:string)  [unwired: 2 in, 1 out]
      n370 = Merge Errors(w814, w816) -> (w817:errorcluster)
      n371 = call "Stop Module.vi"("Origin"=w807) -> ()  [unwired: 10 in, 1 out]
      n372 = call "Error Reported.vi"("Additional Information"=w807, "Error"=w817) -> ()  [unwired: 9 in, 1 out]
    }
  }
  n373 = Merge Errors(w24, w26, w19) -> (w23:errorcluster)
  n374 = call "Close Module.vi"("error in (no error)"=w23, "Module Admin in"=w14) -> ("error out"=w25:errorcluster, "External Launch"=w8:bool, "Module Admin out"=w9:refnum<class "Delacor_lib_QMH_Module Admin.lvclass">)  [unwired: 7 in]
  n375 = Unregister For Events(event registration refnum=w6) -> ()  [unwired: 1 in, 1 out]
  n376 = Unregister For Events(event registration refnum=w13, error in=w25) -> (error out=w22:errorcluster)
  "error out" <- w22
  n377 = case "External Launch?" shown="True" w8 {
    tunnel: w22 -> [_ w818]
    frame False {
    }
    frame True {
      n378 = case shown="No Error" w818 {
        frame No Error {
          n379 = invoke class="VI" method="FP.Close"() -> ()  [unwired: 3 in, 3 out]
        }
        frame Error {
          n380 = invoke on="Invoke Node" class="VI" method="FP.Open"("Activate"=TRUE ("Activate?")) -> ()  [unwired: 4 in, 5 out]
        }
      }
    }
  }
  n381 = local write "Module Admin"(w9) -> ()
